vi "信号光谱11.vi"() -> ()   [LabVIEW 2018]
uses:
  <vilib>/Utility/NIReport.llb/Report Type.ctl
  <vilib>/Utility/file.llb/Write Delimited Spreadsheet (DBL).vi
  <vilib>/Instr/_visa.llb/VISA Configure Serial Port (Instr).vi
  <vilib>/addons/_office/excel.llb/Excel Get Data ([str]).vi
  <vilib>/Utility/NIReport.llb/NI_report.lvclass
  <vilib>/Analysis/NI_AALBase.lvlib
  <vilib>/ptbypt/NI_PtbyPt.lvlib
  <vilib>/Utility/NIReport.llb/NI_ReportGenerationCore.lvlib
  <vilib>/addons/_office/NI_ReportGenerationToolkit.lvlib
  <vilib>/Utility/NIReport.llb/Excel/NI_Excel.lvclass
panel:
  in  "Δy系数（0-1之间）":dbl=1.0 min=0.0 max=1.0
  in  "Δx系数（0-1之间）":dbl=1.0 min=0.0 max=1.0
  out "error out 2":errorcluster
  in  "y初次移动/um":dbl=2.0
  in  "y比例(步/um)":dbl=91.48
  in  "x比例(步/um)":dbl=91.48
  in  "x初次移动/um":dbl=2.0
  in  "运动加速度":i32=200
  in  "运动速度（步数/s）":i32=200
  out "y":i32
  out "x":i32
  out "DeviceKey Out":string
  out "Identification":string
  in  "画面长度（um）":dbl=41.52
  in  "截图等待时间（秒）":u32=10
  in  "y是否取反":bool
  in  "x是否取反":bool
  in  "是否移动光斑":bool
  out "波长范围":dbl[](array[numeric])
  out "Backlight":i32[][](graph)
  in  "?":enum32{"IHR 550", "CCD"}(tab)
  in  "Move To\nTarget Positions":bool
  out "Current UniqueID":string="Mono4"
  in  "Mono ID":string(combo)="Mono1"
  in  "Connect":bool
  out "Initialized JY":bool=TRUE
  in  "Force\nInitialization":bool
  in  "Target Grating":string(combo)="2"
  out "Current Description":string="1" caption="Description"
  out "Grating Index":i32=1
  out "Current Grating":dbl=1200.0
  out "Units":string="nm"
  out "Current WL":dbl=897.9988
  out "Exit Mirror\nPosition":i32(ring)=2 items=["EntranceMirror", "ExitMirror", "Front", "Side"]
  out "Entrance Mirror\nPosition":i32(ring)=2 items=["EntranceMirror", "ExitMirror", "Front", "Side"]
  out "Units 2":string="mm"
  out "Front Entrance":dbl
  in  "Target WL":dbl=2670.0
  in  "Exit Mirror":u16(ring)=3 caption="Target Position Exit Mirror" items=["Front"=2, "Side"=3]
  in  "Entrance Mirror":u16(ring)=2 caption="Target Position\nEntrance Mirror" items=["Front"=2, "Side"=3]
  in  "Target\nFront Entrance":dbl=1.0
  in  "Commande tab":T1(tab)
  in  "Area Number to Display":i32
  in  "Reformat":bool
  in  "GAIN":u16(ring)=2 caption="Device Name" items=["High Light", "Best Dynamic Range", "High Sensitivity"]
  in  "ADC":u16(ring) caption="Device Name" items=["20 kHz       ", " 1 MHz       ", " 1 MHz Ultra "]
  in  "Number of Areas :":u16=1 min=1 step=1
  in  "Integration time (ms) :":i16=30000
  out "Uniques ID":u16(ring) items=["CCD1", "CCD2"]
  in  "Device Name":u16(ring) items=["Synapse CCD (Lateral)", "Synapse_IGA (Axial)"]
  in  "Signal type :":enum16{"TTL Rising Edge", "TTL Falling Edge"}(ring)=enum."TTL Falling Edge"
  in  "Trigger Type :":u16(ring) items=["On Start"=1, "Per Acquisition"=2]
  in  "trigSigTypeString":string
  in  "trigEventString":string
  in  "Enable InputTriggers :":bool
  in  "Number of Cleans":i32=1
  in  "MultiAcqShutterMode":i32(ring)=3 items=["Open For All Spectra"=1, "Open for Each Spectrum"=3]
  in  "Accumulations:":u16=10 min=1 step=1
  in  "Multi Accumulation mode:":bool
  out "Y Pixels:":i32=256
  out "DataSize":i32=1024
  out "X Pixels:":i32=1024
  out "Firmware\nVersion":string="V1.20 CCD_4000"
  out "initialized ?":bool=TRUE
  in  "Continuous":bool
  in  "CCD Busy":bool
  out "indicator":string="Ready !"
  in  "initialize":bool
  in  "ShutterOpen":bool=TRUE caption="Shutter enable"
  in  "Acquire":bool
  in  "Temperature":bool
  in  "Setup":bool
  out "Acq Time(ms)":u32=3401
  in  "Save Backlight":bool
  in  "cut backlight":bool
  out "backlight":bool=TRUE
  in  "是否拟合":bool
  in  "是否保存":bool
  in  "停止程序":bool
  in  "上升下降沿/s":dbl format="%.2p"
  in  "延时/s":dbl format="%.2p"
  in  "占空比/%":dbl=3.0 format="%.2p"
  in  "高电平/V":dbl=4.0 format="%.2p"
  in  "频率/Hz":dbl=6000.0 format="%.3p"
  in  "低电平/V":dbl min=0.0 max=5.0 format="%.2p"
  out "configure error out":errorcluster
  in  "上升下降沿/s 2":dbl format="%.2p"
  in  "上升下降沿 2":i32(ring)=1 items=["上升沿", "下降沿"]
  in  "延时/s 2":dbl format="%.2p"
  in  "占空比/% 2":dbl=3.0 format="%.2p"
  in  "高电平/V 2":dbl=0.002 format="%.2p"
  in  "频率/Hz 2":dbl=6000.0 format="%.3p"
  in  "低电平/V 2":dbl min=0.0 max=5.0 format="%.2p"
  in  "输出信号波形 2":u16(ring) items=["Pulse"]
  in  "设置参数":bool
  out "output control error  4":errorcluster
  in  "低电平持续输出":bool
  in  "Enable":bool
  out "output control error  5":errorcluster
  out "output control error":errorcluster
  out "照明光error out":errorcluster
  in  "照明光VISA":refnum<visa-resource-name>="COM7"
  in  "baud rate":u32=9600 caption="baud rate (115200)" min=9600 max=115200
  in  "data bits (8)":u16=8 min=5 max=8 step=1
  in  "parity (0:none)":enum16{"None", "Odd", "Even", "Mark", "Space"}(ring)
  in  "stop bits (10: 1 bit)":u16(ring)=10 items=["1.0"=10, "1.5"=15, "2.0"=20]
  out "Δw2>C":bool=TRUE
  in  "C=w-w0":dbl=2.0 format="%#_13g"
  out "θi":dbl
  out "Δw1>C":bool=TRUE
  in  "角度倍乘系数":dbl=1.5
  in  "w0":dbl format="%#_13g"
  out "Spectrum":cluster{"Y":dbl[], "Y":dbl[]}[](graph)
  out "拟合参数":dbl[](array[numeric])
  out "xc":dbl
  out "w":dbl
  out "范围内？":bool[](array[boolean])
  in  "滤波阈值":dbl=3000.0 format="%#_13g"
  out "最终存储路径":path
  out "angle":dbl
  out "图片地址":string
  in  "开光时间/ms":u32=50
  out "正在测量":bool
  in  "终止测量":bool
  out "结果展示":dbl[][](array[numeric])=[[37.33100777239877, 2672.955043835526, 29.54153292599307, 222755.0, 50.0], [37.36593979472361, 2672.656498058864, 30.113284142729572, 222833.0, 50.0], [38.96986225690859, 2673.3337152325566, 33.38805102415213, 222910.0, 75.0], [37.39946104045098, 2676.4005085744548, 31.215565446104666, 222948.0, 47.0], [35.862209164247574, 2671.7826876859012, 30.355582265151796, 223028.0, 47.0]]
  in  "测量次数":i32=1
  in  "开始测量":bool
  in  "照明光":bool
  in  "Enable 2":bool
  out "Output 2":bool
  in  "上升下降沿":i32(ring)=1 items=["上升沿", "下降沿"]
  in  "channel输出口":i32(ring) items=["Channel 1", "Channel 2"]
  in  "输出信号波形":u16(ring) items=["Pulse"]
  out "output control error 2":errorcluster
  out "Output":bool
  in  "VISA 信号发生器":refnum<visa-resource-name>="USB0::0x1AB1::0x0641::DG4E192200870::INSTR"
  out "error out":errorcluster
  out "Gratings":dbl[](array[numeric])=[1200.0, 300.0]
  out "Data":i32[][](graph)
  out "trigAddress":i32
  out "Gain Number":i32[](array[numeric])=[10, 11, 12, 13, 8, 2]
  out "ADC Number":i32[](array[numeric])=[0, 1, 2, 3, 4]
  out "temp graph":dbl(graph)=-134.538067
  in  "Close":bool=TRUE
  out "JYCCDLib.IJYCCDReqd":refnum<k7>
  out "areas :":i32[][](array[numeric])=[[1], [1], [1], [1024], [256], [1], [256]]
  out "best fit":cluster{"Y":dbl[], "Y":dbl[]}[](graph)
  in  "拟合起点":i32=200
  in  "拟合终点":i32=850
  out "最终存储路径 2":path
  in  "Constante de condition\n(Voir l'aide contextuelle)":bool
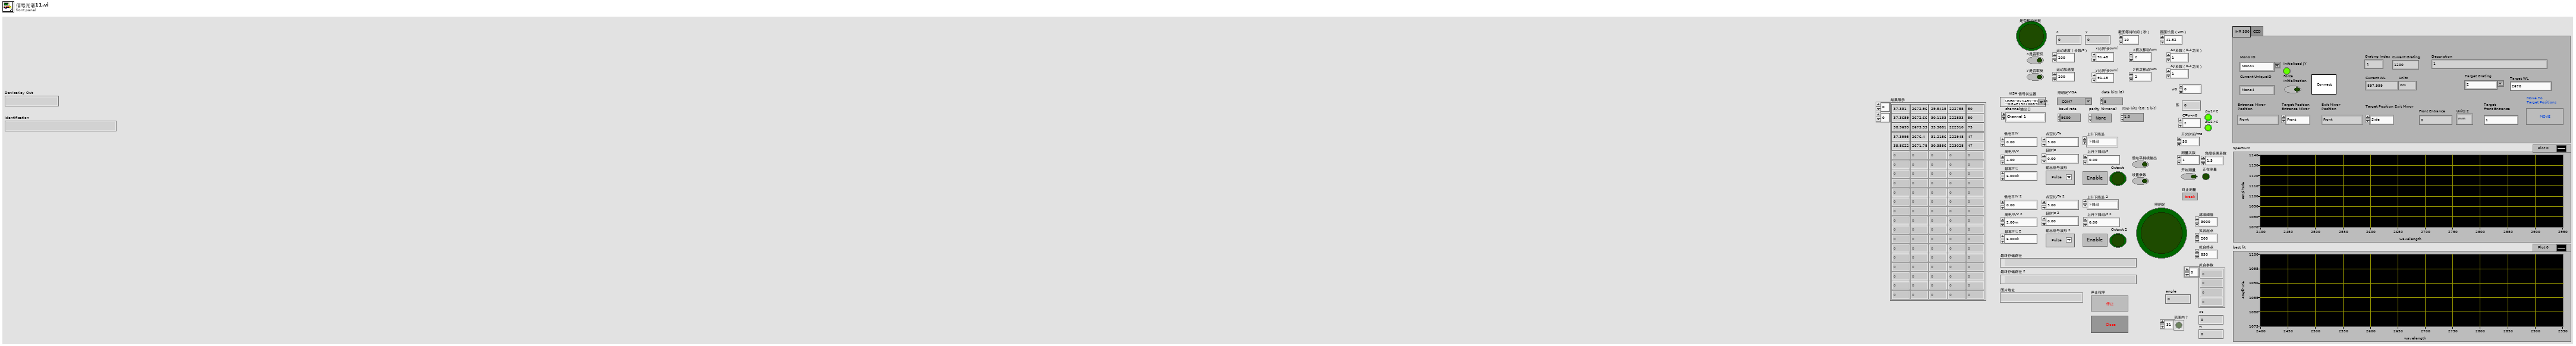
[diagram p1: front panel]
types:
  T1 = enum32{"Settings", "Trigger In", "Multi-Accu.", "Infos"}
  T2 = enum8{"Enabled", "Disabled", "Disabled and Grayed Out"}
  T3 = enum16{"maximized", "minimized", "normal", "no change"}
  T4 = typedef "NI_ReportGenerationCore.lvlib/Report Type.ctl" = enum16{"HTML", "Word", "Excel"}
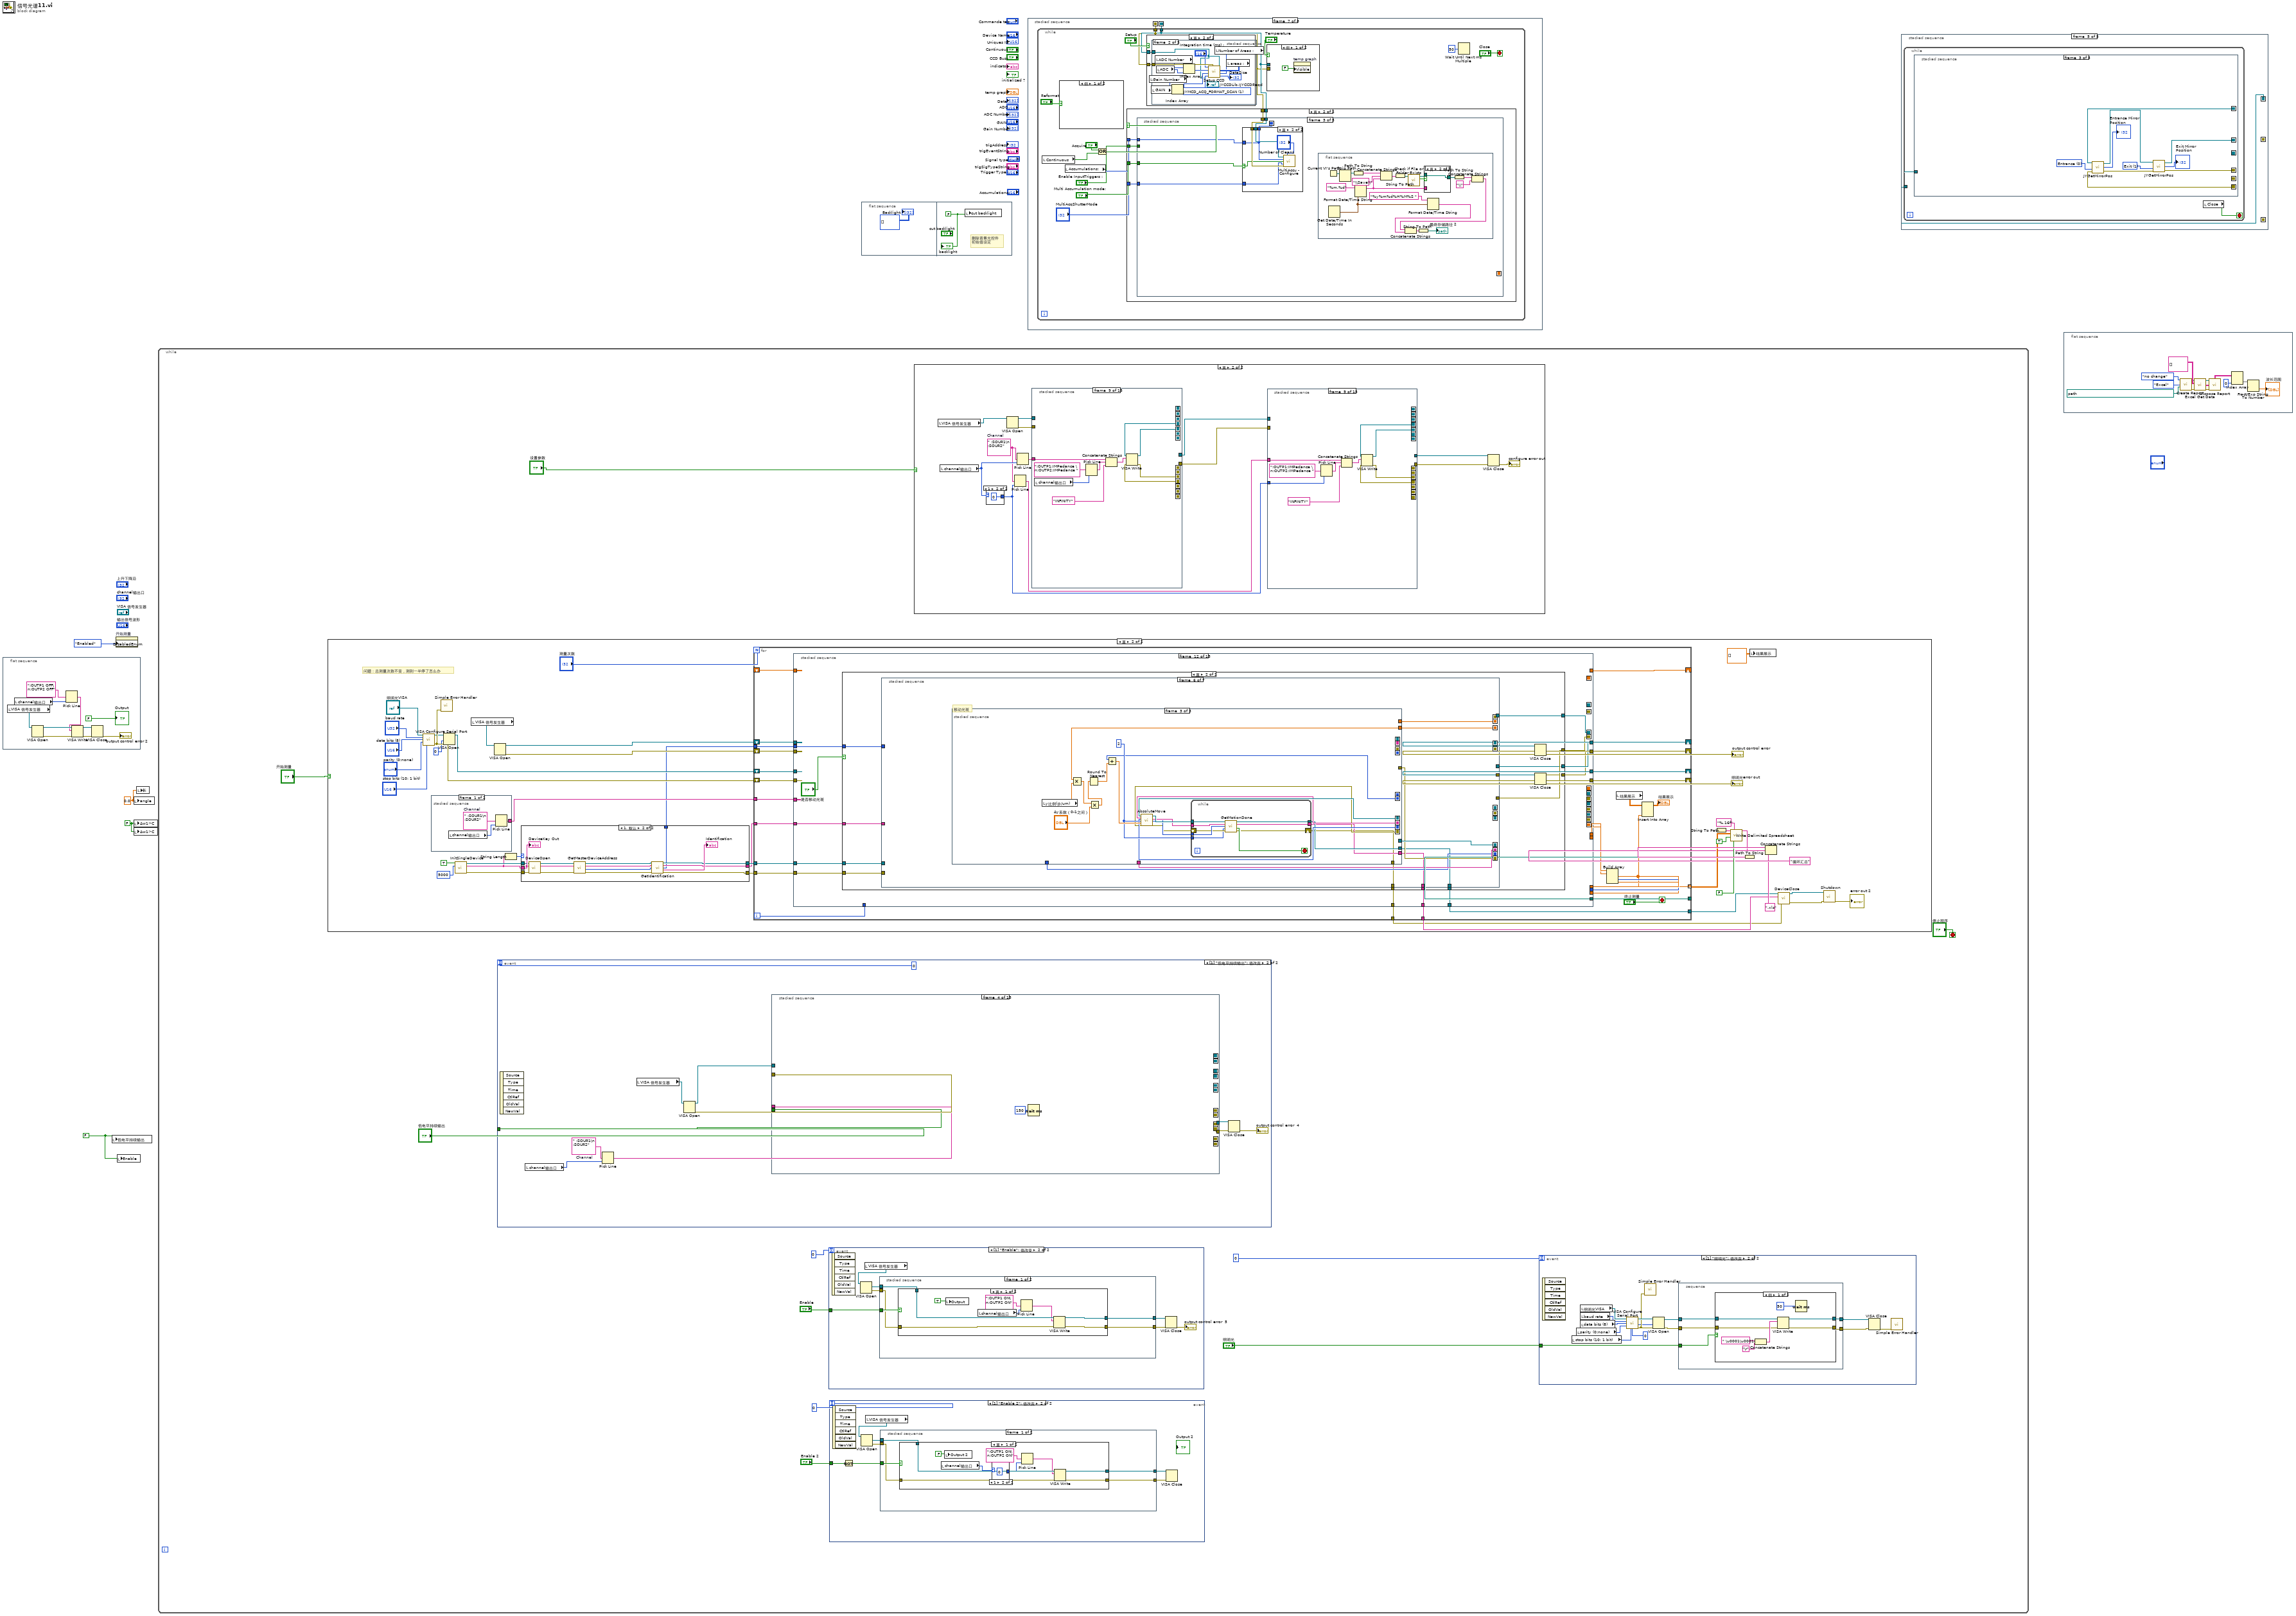
[diagram p0: block diagram]
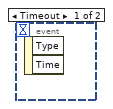
[diagram p2: hidden frame]
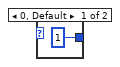
[diagram p3: hidden frame]
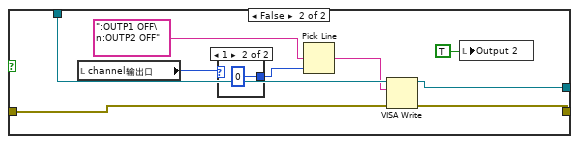
[diagram p4: hidden frame]
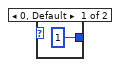
[diagram p5: hidden frame]
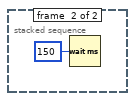
[diagram p6: hidden frame]
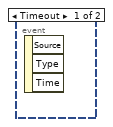
[diagram p7: hidden frame]
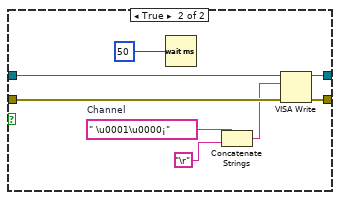
[diagram p8: hidden frame]
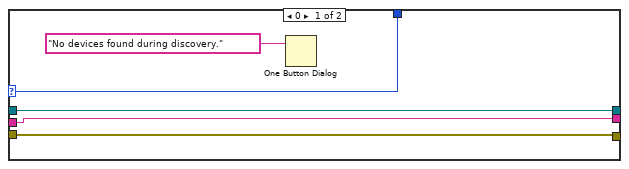
[diagram p10: hidden frame]
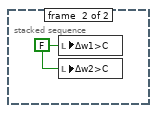
[diagram p11: hidden frame]
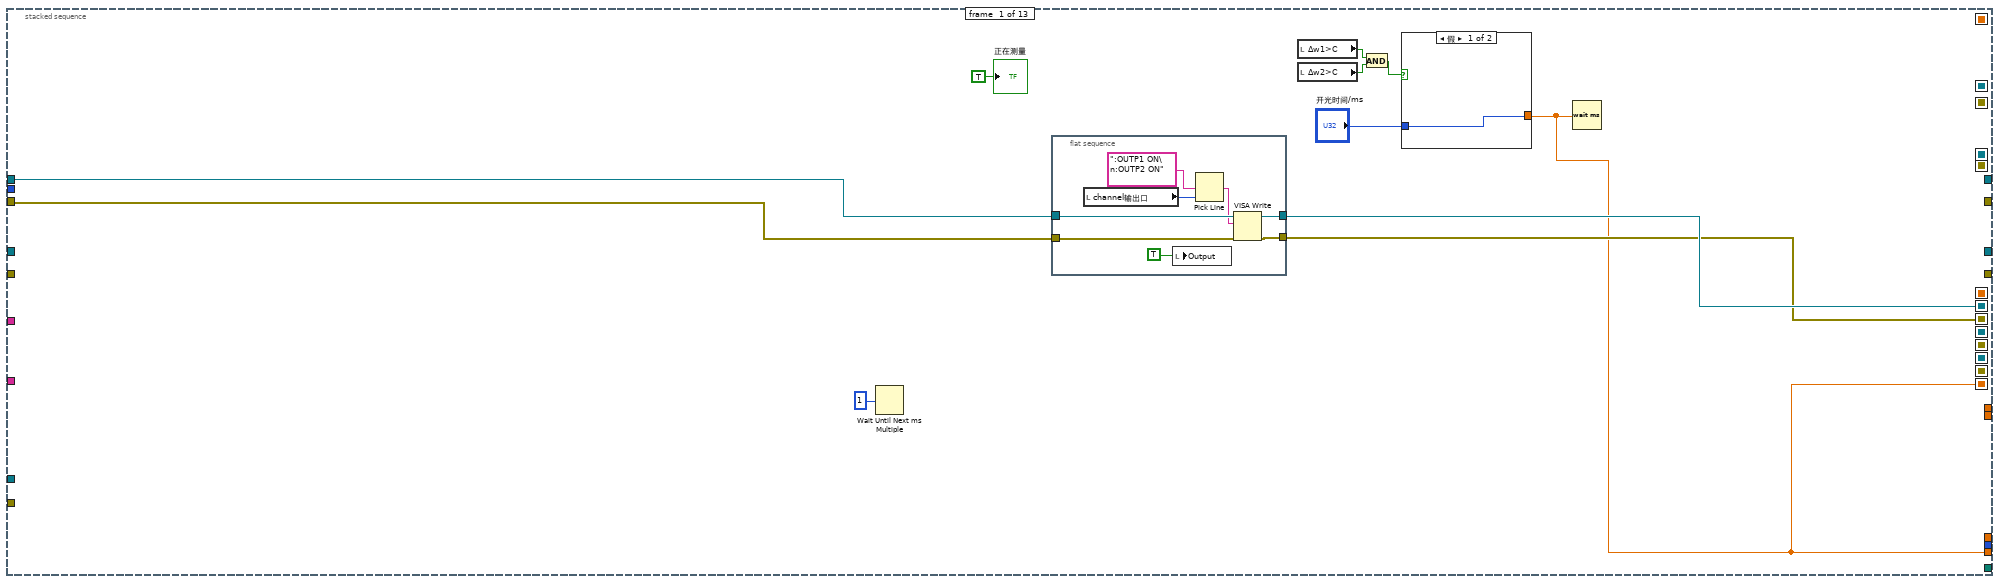
[diagram p12: hidden frame]
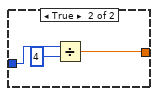
[diagram p13: hidden frame]
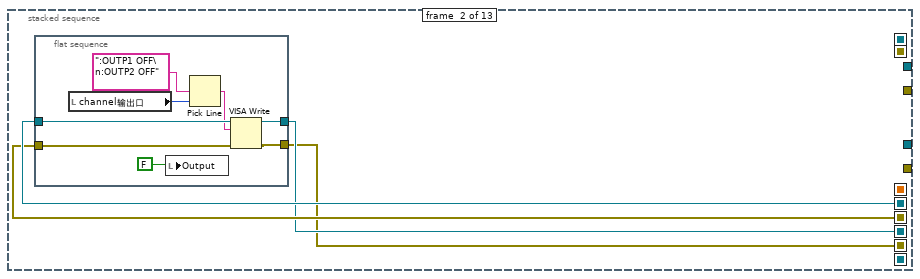
[diagram p14: hidden frame]
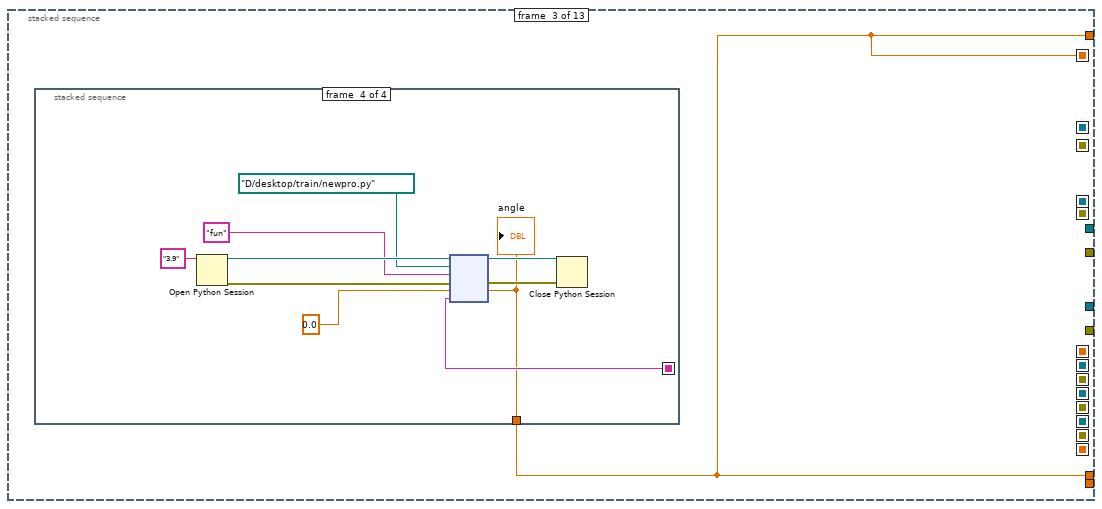
[diagram p15: hidden frame]
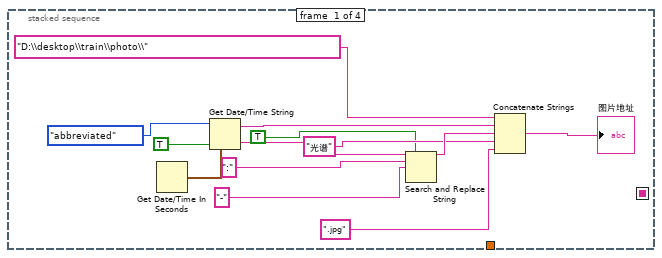
[diagram p16: hidden frame]
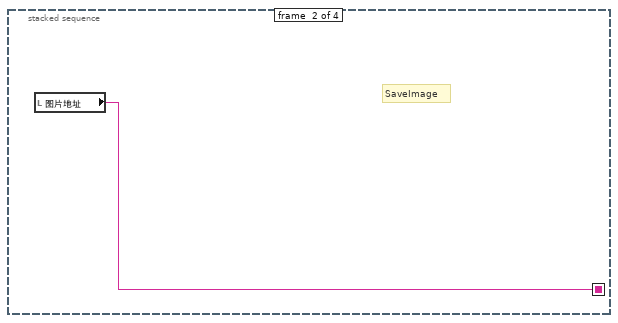
[diagram p17: hidden frame]
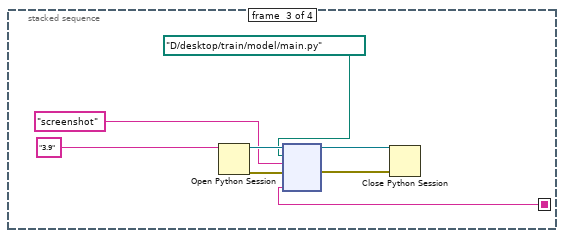
[diagram p18: hidden frame]
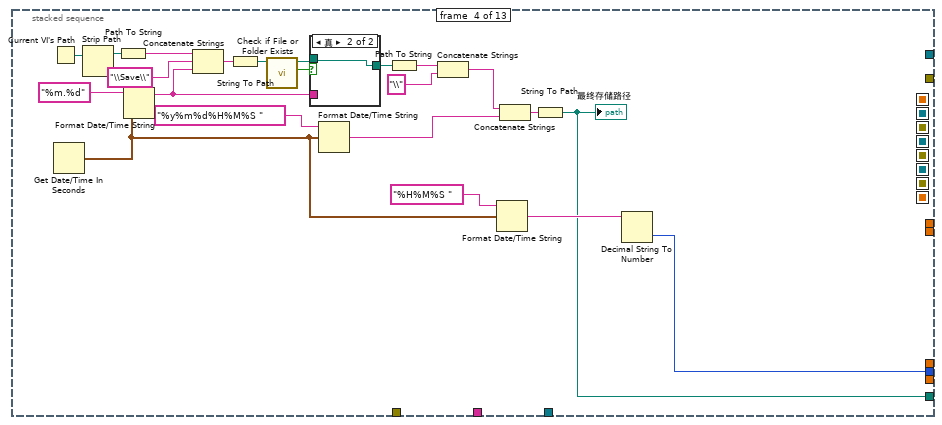
[diagram p19: hidden frame]
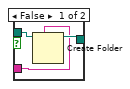
[diagram p20: hidden frame]
diagram:
  w2 = FALSE ("Δw1>C")
  w3 = 0.0 ("angle")
  w1 = FALSE
  n1 = flat-sequence {
    frame #0 {
      n2 = local read "VISA 信号发生器"() -> (w8:refnum<visa-resource-name>)
      n3 = local read "channel输出口"() -> (w6:i32)
      n4 = VISA Open(VISA resource name=w8) -> (VISA resource name=w14:refnum<visa-resource-name>, error out=w13:errorcluster)  [unwired: 4 in]
      n5 = Pick Line(multi-line string=":OUTP1 OFF\n:OUTP2 OFF" ("write buffer"), line index=w6) -> (output string=w5:string)  [unwired: 1 in]
      n6 = VISA Write(VISA resource name=w14, write buffer=w5, error in (no error)=w13) -> (VISA resource name out=w11:refnum<visa-resource-name>, error out=w10:errorcluster)  [unwired: 1 out]
      n7 = VISA Close(VISA resource name=w11, error in (no error)=w10) -> (error out=→"output control error 2":errorcluster)
      "Output" <- FALSE ("布尔")
    }
  }
  n8 = local write "低电平持续输出"(w1) -> ()
  n9 = property on="开始测量" class="Bool"("DisabledEnum"=T2."Enabled" ("禁用")) -> ()  [unwired: 2 in, 2 out]
  n10 = local write "Enable"(w1) -> ()
  n11 = local write "angle"(w3) -> ()
  n12 = local write "Δw1>C"(w2) -> ()
  n13 = local write "Δw1>C"(w2) -> ()
  n14 = local write "θi"(w3) -> ()
  n15 = while {
    stop <- "停止程序" stop-if-true
    n16 = case shown="真" "开始测量" {
      frame False {
      }
      frame True {
        # "问题：总测量次数不变，测到一半停了怎么办"
        n17 = call-poly "VISA Configure Serial Port"("VISA resource name"="照明光VISA", "baud rate (9600)"="baud rate", "data bits (8)"="data bits (8)", "parity (0:none)"="parity (0:none)", "stop bits (10: 1 bit)"="stop bits (10: 1 bit)") -> ("VISA resource name out"=w134:refnum<visa-resource-name>, "error out"=w135:errorcluster)  [unwired: 9 in]
        n18 = stacked-sequence {
          tunnel: [w164 _] -> w138
          frame #0 {
            w165 = " :SOUR1\n :SOUR2"  # Channel
            n19 = local read "channel输出口"() -> (w166:i32)
            n20 = Pick Line(multi-line string=w165, line index=w166) -> (output string=w164:string)  [unwired: 1 in]
          }
          frame #1 {
            w167 = FALSE ("Δw1>C")
            n21 = local write "Δw1>C"(w167) -> ()
            n22 = local write "Δw2>C"(w167) -> ()
          }
        }
        n23 = call <vilib>:"Simple Error Handler.vi"("error in (no error)"=w135) -> ()  [unwired: 4 in, 5 out]
        n24 = VISA Open(access mode=0, error in (no error)=w135, VISA resource name=w134) -> (VISA resource name=w127:refnum<visa-resource-name>, error out=w126:errorcluster)  [unwired: 2 in]
        n25 = call "InitSingleDevice.vi"("msecDelayForDiscovery"=5000, "logging"=TRUE) -> ("error out"=w107:errorcluster, "DeviceKey Out"=w106:string, "CmdLib Out"=w108:refnum<k24>)  [unwired: 3 in]
        n26 = local read "VISA 信号发生器"() -> (w143:refnum<visa-resource-name>)
        n27 = VISA Open(VISA resource name=w143) -> (VISA resource name=w142:refnum<visa-resource-name>, error out=w141:errorcluster)  [unwired: 4 in]
        n28 = String Length(string=w106) -> (length=w109:i32)
        n29 = case shown="1, 默认" w109 {
          selector: w109 -> [w144 _]
          tunnel: w108 -> [w147 w154]
          tunnel: w107 -> [w146 w158]
          tunnel: w106 -> [w145 w156]
          tunnel: [w147 w152] -> w105
          tunnel: [w146 w151] -> w103
          tunnel: [w145 w150] -> w104
          tunnel: [w144 w149] -> w102
          frame 0 {
            n30 = One Button Dialog(message="No devices found during discovery.") -> ()  [unwired: 1 in, 1 out]
          }
          frame 1, Default {
            n31 = call "DeviceOpen.vi"("error in (no error)"=w158, "DeviceKey In"=w156, "CmdLib In"=w154) -> ("error out"=w157:errorcluster, "DeviceKey Out"=w155:string, "CmdLib Out"=w153:refnum<k24>)  [unwired: 2 in]
            n32 = call "GetMasterDeviceAddress.vi"("error in (no error)"=w157, "DeviceKey In"=w155, "CmdLib In"=w153) -> ("error out"=w161:errorcluster, "Device Address"=w162:i32, "DeviceKey Out"=w159:string, "CmdLib Out"=w160:refnum<k24>)  [unwired: 1 in]
            n33 = call "GetIdentification.vi"("CmdLib In"=w160, "DeviceKey In"=w159, "Device Address In"=w162, "error in (no error)"=w161) -> ("CmdLib Out"=w152:refnum<k24>, "DeviceKey Out"=w150:string, "Device Address Out"=w149:i32, "Identification"=→"Identification":string, "error out"=w151:errorcluster)  [unwired: 7 in]
            "DeviceKey Out" <- w156
          }
        }
        n34 = for {
          N: "测量次数" -> [_]
          tunnel: w138 -> [w194]
          shift-right: [w190] -> w137
          shift-left: w142 -> [w196]
          shift-right: [w189] -> w136
          shift-left: w141 -> [w195]
          shift-right: [w188] -> w140
          shift-left: w127 -> [w193]
          shift-right: [w187] -> w139
          shift-left: w126 -> [w192]
          tunnel: [w177] -> w116 mode=indexing
          shift-right: [w182] -> _
          shift-left: _ -> [w181]
          tunnel: [w178] -> w113
          tunnel: w105 -> [w174]
          tunnel: w104 -> [w173]
          tunnel: w103 -> [w172]
          tunnel: w102 -> [w171]
          tunnel: [w170] -> w101
          tunnel: [w169] -> w100
          tunnel: [w168] -> w99
          i -> [w180]
          stop <- "终止测量" stop-if-true
          n35 = stacked-sequence {
            seq-local: [w203 _ _ _ _ _ _ _ _ _ _ _ _] -> [_ w223 _ _ _ _ _ _ _ _ _ _ _]
            seq-local: [w202 _ _ _ _ _ _ _ _ _ _ _ _] -> [_ w222 _ _ _ _ _ _ _ _ _ _ _]
            seq-local: [_ _ _ _ _ w308 _ _ _ _ _ _ _] -> [_ _ _ _ _ _ _ _ w426 _ _ _ _]
            seq-local: [_ _ _ _ _ w307 _ _ _ _ _ _ _] -> [_ _ _ _ _ _ _ _ w427 _ _ _ _]
            seq-local: [_ w221 _ _ _ _ _ _ _ _ _ _ _] -> [_ _ _ _ w294 _ _ _ _ _ _ _ _]
            seq-local: [_ w220 _ _ _ _ _ _ _ _ _ _ _] -> [_ _ _ _ w293 _ _ _ _ _ _ _ _]
            seq-local: [_ _ _ _ w292 _ _ _ _ _ _ _ _] -> [_ _ _ _ _ _ _ w410 _ _ _ _ _]
            seq-local: [_ _ _ _ w291 _ _ _ _ _ _ _ _] -> [_ _ _ _ _ _ _ w409 _ _ _ _ _]
            seq-local: [_ _ w232 _ _ _ _ _ _ _ _ _ _] -> [_ _ _ _ _ _ _ _ _ _ w436 _ _]
            seq-local: [_ _ _ _ _ _ w317 _ _ _ _ _ _] -> [_ _ _ _ _ _ _ _ _ _ w431 _ _]
            seq-local: [w197 _ _ _ _ _ _ _ _ _ _ _ _] -> [_ _ _ _ _ _ w315 _ _ _ _ _ _]
            seq-local: [_ _ _ _ _ _ _ w407 _ _ _ _ _] -> [_ _ _ _ _ _ _ _ _ _ _ w505 _]
            seq-local: [_ _ _ _ _ _ _ w408 _ _ _ _ _] -> [_ _ _ _ _ _ _ _ _ _ _ w504 _]
            tunnel: w196 -> [w205 _ _ _ _ _ _ _ _ _ _ _ _]
            tunnel: w195 -> [w204 _ _ _ _ _ _ _ _ _ _ _ _]
            tunnel: [_ _ _ _ _ _ _ _ _ _ _ w503 _] -> w190
            tunnel: [_ _ _ _ _ _ _ _ _ _ _ w502 _] -> w189
            tunnel: w194 -> [_ _ _ _ _ _ _ _ _ _ _ _ _]
            tunnel: w193 -> [_ _ _ _ _ w311 _ _ _ _ _ _ _]
            tunnel: w192 -> [_ _ _ _ _ w310 _ _ _ _ _ _ _]
            tunnel: [_ _ _ _ _ _ _ _ w423 _ _ _ _] -> w188
            tunnel: [_ _ _ _ _ _ _ _ w422 _ _ _ _] -> w187
            tunnel: [_ _ w232 _ _ _ _ _ _ _ _ _ _] -> w186
            tunnel: [_ _ _ _ _ _ w318 _ _ _ _ _ _] -> w185
            tunnel: [_ _ _ _ _ _ w317 _ _ _ _ _ _] -> w184
            tunnel: [_ _ _ w266 _ _ _ _ _ _ _ _ _] -> w183
            tunnel: [w197 _ _ _ _ _ _ _ _ _ _ _ _] -> w179
            tunnel: [_ _ w232 _ _ _ _ _ _ _ _ _ _] -> w182
            tunnel: w181 -> [_ _ _ _ _ _ _ _ _ _ w435 _ _]
            tunnel: w180 -> [_ _ _ _ _ _ _ _ _ _ w433 _ _]
            tunnel: [_ _ _ w265 _ _ _ _ _ _ _ _ _] -> w178
            tunnel: w174 -> [_ _ _ _ _ _ _ _ _ _ _ w501 _]
            tunnel: w173 -> [_ _ _ _ _ _ _ _ _ _ _ w500 _]
            tunnel: w172 -> [_ _ _ _ _ _ _ _ _ _ _ w499 _]
            tunnel: w171 -> [_ _ _ _ _ _ _ _ _ _ _ w498 _]
            tunnel: [_ _ _ _ _ _ _ _ _ _ _ w497 _] -> w170
            tunnel: [_ _ _ _ _ _ _ _ _ _ _ w496 _] -> w169
            tunnel: [_ _ _ _ _ _ _ _ _ _ _ w495 _] -> w168
            frame #0 {
              n36 = Wait Until Next ms Multiple(millisecond multiple=u32 1 ("毫秒倍数")) -> ()  [unwired: 1 out]
              n37 = flat-sequence {
                tunnel: w205 -> [w219]
                tunnel: w204 -> [w218]
                tunnel: [w213] -> w203
                tunnel: [w212] -> w202
                frame #0 {
                  n38 = local read "channel输出口"() -> (w215:i32)
                  n39 = local write "Output"(TRUE ("布尔")) -> ()
                  n40 = Pick Line(multi-line string=":OUTP1 ON\n:OUTP2 ON" ("write buffer"), line index=w215) -> (output string=w214:string)  [unwired: 1 in]
                  n41 = VISA Write(VISA resource name=w219, write buffer=w214, error in (no error)=w218) -> (VISA resource name out=w213:refnum<visa-resource-name>, error out=w212:errorcluster)  [unwired: 1 out]
                }
              }
              n42 = local read "Δw1>C"() -> (w199:bool)
              n43 = local read "Δw2>C"() -> (w200:bool)
              n44 = And(x=w199, y=w200) -> (x .and. y?=w198:bool)
              n45 = case shown="假" w198 {
                tunnel: [w208 w209] -> w197
                tunnel: "开光时间/ms" -> [w208 w211]
                frame False {
                }
                frame True {
                  n46 = Divide(x=w211, y=u32 4) -> (x/y=w209:dbl)
                }
              }
              n47 = Wait (ms)(milliseconds to wait=w197) -> ()  [unwired: 1 out]
              "正在测量" <- TRUE
            }
            frame #1 {
              n48 = flat-sequence {
                tunnel: w223 -> [w231]
                tunnel: w222 -> [w230]
                tunnel: [w225] -> w221
                tunnel: [w224] -> w220
                frame #0 {
                  n49 = local read "channel输出口"() -> (w227:i32)
                  n50 = local write "Output"(FALSE ("布尔")) -> ()
                  n51 = Pick Line(multi-line string=":OUTP1 OFF\n:OUTP2 OFF" ("write buffer"), line index=w227) -> (output string=w226:string)  [unwired: 1 in]
                  n52 = VISA Write(VISA resource name=w231, write buffer=w226, error in (no error)=w230) -> (VISA resource name out=w225:refnum<visa-resource-name>, error out=w224:errorcluster)  [unwired: 1 out]
                }
              }
            }
            frame #2 {
              n53 = stacked-sequence {
                seq-local: [_ w246 _ _] -> [_ _ w247 w256]
                tunnel: [_ _ _ w255] -> w232
                frame #0 {
                  n54 = Get Date/Time In Seconds() -> (seconds since 1Jan1904=w242:timestamp)
                  n55 = Get Date/Time String(date format (0)=enum16{"short", "long", "abbreviated"}."abbreviated" ("日期格式(0)"), seconds (now)=w242, want seconds? (F)=TRUE ("需要秒？(F)")) -> (date string=w245:string, time string=w243:string)
                  n56 = Search and Replace String(replace all?=TRUE ("替换全部？(F)"), input string=w243, search string=":" ("搜索字符串"), replace string="-" ("替换字符串(\"\")")) -> (result string=w244:string)  [unwired: 4 in, 3 out]
                  n57 = Concatenate Strings("D:\\desktop\\train\\photo\\", w245, w244, "光谱" ("字符串"), ".jpg" ("字符串")) -> (→"图片地址":string)
                }
                frame #1 {
                  # "SaveImage"
                  n58 = local read "图片地址"() -> (w246:string)
                }
                frame #2 {
                  n59 = Open Python Session(python version="3.9" ("Python version")) -> (session out=w254:refnum<k35>, error out=w252:errorcluster)  [unwired: 2 in]
                  n60 = node(w254, path "D:/desktop/train/model/main.py" ("module path"), "screenshot" ("function name"), w252, w247) -> (w253:refnum<k35>, w251:errorcluster)  [unwired: 3 in, 2 out]
                  n61 = Close Python Session(session in=w253, error in=w251) -> ()  [unwired: 1 out]
                }
                frame #3 {
                  n62 = Open Python Session(python version="3.9" ("Python version")) -> (session out=w263:refnum<k35>, error out=w261:errorcluster)  [unwired: 2 in]
                  n63 = node(w263, path "D:/desktop/train/newpro.py" ("module path"), "fun" ("function name"), w261, 0.0, w256) -> (w262:refnum<k35>, w260:errorcluster, w255:dbl)  [unwired: 1 in, 2 out]
                  "angle" <- w255
                  n64 = Close Python Session(session in=w262, error in=w260) -> ()  [unwired: 1 out]
                }
              }
            }
            frame #3 {
              n65 = Current VI's Path() -> (path=w275:path)
              n66 = Get Date/Time In Seconds() -> (seconds since 1Jan1904=w268:timestamp)
              n67 = Strip Path(path=w275) -> (stripped path=w276:path)  [unwired: 1 out]
              n68 = Path To String(path=w276) -> (string=w277:string)
              n69 = Format Date/Time String(time format string (%c)="%m.%d" ("时间格式字符串(%c)"), seconds (now)=w268) -> (date/time string=w283:string)  [unwired: 1 in]
              n70 = Concatenate Strings(w277, "\\Save\\" ("字符串"), w283) -> (w278:string)
              n71 = String To Path(string=w278) -> (path=w279:path)
              n72 = call <vilib>:"Check if File or Folder Exists.vi"("path"=w279) -> ("file or folder exists?"=w280:bool, "dup path"=w282:path)  [unwired: 8 in, 1 out]
              n73 = case shown="真" w280 {
                tunnel: [w289 w290] -> w281
                tunnel: w282 -> [w288 w290]
                tunnel: w283 -> [w287 _]
                frame False {
                  n74 = Create Folder(prompt (Create Folder)=w287, path (use dialog)=w288) -> (created path=w289:path)  [unwired: 1 in, 2 out]
                }
                frame True {
                }
              }
              n75 = Format Date/Time String(time format string (%c)="%y%m%d%H%M%S " ("时间格式字符串(%c)"), seconds (now)=w268) -> (date/time string=w286:string)  [unwired: 1 in]
              n76 = Path To String(path=w281) -> (string=w284:string)
              n77 = Concatenate Strings(w284, "\\" ("字符串")) -> (w285:string)
              n78 = Format Date/Time String(time format string (%c)="%H%M%S " ("时间格式字符串(%c)"), seconds (now)=w268) -> (date/time string=w267:string)  [unwired: 1 in]
              n79 = Concatenate Strings(w285, w286) -> (w274:string)
              n80 = String To Path(string=w274) -> (path=w265:path)
              "最终存储路径" <- w265
              n81 = Decimal String To Number(string=w267) -> (number=w266:i32)  [unwired: 2 in, 1 out]
            }
            frame #4 {
              n82 = flat-sequence {
                tunnel: w294 -> [w303]
                tunnel: w293 -> [w302]
                tunnel: [w298] -> w292
                tunnel: [w297] -> w291
                frame #0 {
                  n83 = local read "channel输出口"() -> (w296:i32)
                  n84 = case shown="1" w296 {
                    tunnel: [1 0] -> w295
                    frame 0, Default {
                    }
                    frame 1 {
                    }
                  }
                  n85 = local write "Output 2"(FALSE ("布尔")) -> ()
                  n86 = Pick Line(multi-line string=":OUTP1 OFF\n:OUTP2 OFF" ("write buffer"), line index=w295) -> (output string=w299:string)  [unwired: 1 in]
                  n87 = VISA Write(VISA resource name=w303, write buffer=w299, error in (no error)=w302) -> (VISA resource name out=w298:refnum<visa-resource-name>, error out=w297:errorcluster)  [unwired: 1 out]
                }
              }
            }
            frame #5 {
              w306 = " \u0001\u0001¢"  # Channel
              n88 = Wait (ms)(milliseconds to wait=500) -> ()  [unwired: 1 out]
              n89 = Concatenate Strings(w306, "\r") -> (w312:string)
              n90 = local write "照明光"(FALSE ("照明光")) -> ()
              n91 = VISA Write(VISA resource name=w311, write buffer=w312, error in (no error)=w310) -> (VISA resource name out=w308:refnum<visa-resource-name>, error out=w307:errorcluster)  [unwired: 1 out]
            }
            frame #6 {
              n92 = local read "Area Number to Display"() -> (w360:i32)
              n93 = local read "JYCCDLib.IJYCCDReqd"() -> (w356:refnum<k7>)
              n94 = Get Date/Time In Seconds() -> (seconds since 1Jan1904=w369:timestamp)
              n95 = local read "最终存储路径"() -> (w383:path)
              n96 = Get Date/Time String(date format (0)=enum16{"short", "long", "abbreviated"}."abbreviated" ("日期格式(0)"), seconds (now)=w369, want seconds? (F)=TRUE ("需要秒？(F)")) -> (date string=w377:string, time string=w372:string)
              n97 = call "MultiAccu - Acquire spectral.vi"("error in"=errorcluster {"status"=FALSE, "code"=0, "source"=""}, "Accumulations:"=u16 1, "ShutterOpen"=TRUE, "JYCCDLib.IJYCCDReqd"=w356) -> ("Acq Time(ms)"=w362:u32, "Array Out"=w361:i32[][][])  [unwired: 1 out]
              n98 = local write "Acq Time(ms)"(w362) -> ()
              n99 = local read "cut backlight"() -> (w344:bool)
              n100 = local read "backlight"() -> (w342:bool)
              n101 = Search and Replace String(replace all?=TRUE ("替换全部？(F)"), input string=w372, search string=":" ("搜索字符串"), replace string="-" ("替换字符串(\"\")")) -> (result string=w376:string)  [unwired: 4 in, 3 out]
              n102 = Path To String(path=w383) -> (string=w366:string)
              n103 = And(x=w344, y=w342) -> (x .and. y?=w343:bool)
              n104 = call "Array reset dimension.vi"("Area Number"=w360, "Array In"=w361) -> ("Array Out"=w346:i32[][])
              n105 = Concatenate Strings(w366, w377, w376, "光谱" ("字符串"), ".xls" ("字符串")) -> (w381:string)
              n106 = case shown="真" w343 {
                tunnel: [w403 w405] -> w345
                tunnel: w346 -> [w403 w404]
                frame False {
                }
                frame True {
                  n107 = local read "Backlight"() -> (w406:i32[][])
                  n108 = Subtract(x=w404, y=w406) -> (x-y=w405:i32[][])
                }
              }
              n109 = String To Path(string=w381) -> (path=w382:path)
              n110 = local write "Data"(w346) -> ()
              n111 = local read "波长范围"() -> (w323:dbl[])
              n112 = Index Array(array=w345, index (row)=0 ("索引 (行)")) -> (element=w384:i32[])  [unwired: 1 in]
              n113 = Reverse 1D Array(array=w384) -> (reversed array=w320:i32[])
              n114 = local read "angle"() -> (w322:dbl)
              n115 = local read "拟合起点"() -> (w332:i32)
              n116 = local read "拟合终点"() -> (w334:i32)
              n117 = call <vilib>:"Median Filter.vi"("left rank"=6, "X"=w320) -> ("Filtered X"=w319:dbl[])  [unwired: 8 in, 1 out]
              n118 = Build Array(w322, w315, 0.0 ("元素")) -> (w321:dbl[])
              n119 = Subtract(x=w334, y=w332) -> (x-y=w331:i32)
              n120 = call "Convert to Dynamic Data"("Array"=w323) -> ("Dynamic Data Type"=w353:dynamicdata)  [unwired: 3 in]
              n121 = call "Convert to Dynamic Data2"("Array"=w320) -> ("Dynamic Data Type"=w352:dynamicdata)  [unwired: 3 in]
              n122 = Array Subset(array=w323, index=w332, length=w331) -> (w329:dbl[])
              n123 = call "Build XY Graph2"("Y Input"=w352, "X Input"=w353) -> ("XY Graph"=→"Spectrum":cluster{"Y":dbl[], "Y":dbl[]}[])  [unwired: 8 in, 1 out]
              n124 = call "转换至动态数据6"("Array"=w329) -> ("Dynamic Data Type"=w350:dynamicdata)  [unwired: 3 in]
              n125 = In Range and Coerce(upper limit="滤波阈值", x=w319, lower limit=-100.0) -> (In Range?=w337:bool[])  [unwired: 1 out]
              "范围内？" <- w337
              n126 = Not(x=w337) -> (.not. x?=w336:bool[])
              n127 = Or Array Elements(Boolean array=w336) -> (logical OR=w339:bool)
              n128 = local read "X Pixels:"() -> (w338:i32)
              n129 = local read "波长范围"() -> (w324:dbl[])
              n130 = local read "滤波阈值"() -> (w335:dbl)
              n131 = case shown="真" w339 {
                tunnel: w338 -> [_ w390]
                tunnel: w319 -> [w386 w389]
                tunnel: [w386 w388] -> w330
                tunnel: w335 -> [_ w387]
                frame False {
                }
                frame True {
                  n132 = for {
                    N: w390 -> [_]
                    tunnel: w389 -> [w394] mode=indexing
                    tunnel: [w393] -> w388 mode=indexing
                    shift-right: [w393] -> _
                    shift-left: _ -> [w392]
                    tunnel: w387 -> [w391]
                    n133 = Greater?(x=w394, y=w391) -> (0:w396:bool)
                    n134 = Less?(x=w394, y=-100.0) -> (x < y?=w397:bool)
                    n135 = Or(x=w396, y=w397) -> (x .or. y?=w395:bool)
                    n136 = case shown="真" w395 {
                      tunnel: w394 -> [w399 _]
                      tunnel: [w399 w401] -> w393
                      tunnel: w392 -> [_ w402]
                      frame False {
                      }
                      frame True {
                        n137 = call <vilib>:"Median Filter PtByPt.vi"("rank"=5, "x"=w402) -> ("Filtered x"=w401:dbl)  [unwired: 2 in, 1 out]
                      }
                    }
                  }
                }
              }
              n138 = Array Subset(array=w330, index=w332, length=w331) -> (w333:dbl[])
              n139 = call "转换至动态数据5"("Array"=w333) -> ("Dynamic Data Type"=w351:dynamicdata)  [unwired: 3 in]
              n140 = call "曲线拟合2"("Locations"=w350, "Signals"=w351) -> ("best fit"=w355:dynamicdata, "non-linear coefficients"=w354:dynamicdata)  [unwired: 5 in, 3 out]
              n141 = call "从动态数据转换3"("Dynamic Data Type"=w354) -> ("Array"=w347:dbl[])  [unwired: 3 in]
              "拟合参数" <- w347
              n142 = call "从动态数据转换4"("Dynamic Data Type"=w355) -> ("Array"=w328:dbl[])  [unwired: 3 in]
              n143 = Build Array(w323, w319, w328, w347, w321) -> (w385:dbl[][])
              n144 = call-poly <vilib>:"Write Delimited Spreadsheet.vi"("file path (dialog if empty)"=w382, "format (%.3f)"="%.16f", "2D data"=w385, "append to file? (new file:F)"=TRUE ("append to file? (F)"), "transpose? (no:F)"=TRUE ("transpose? (F)")) -> ()  [unwired: 9 in, 2 out]
              n145 = Index Array(array=w347, index #1=0 ("索引"), index #2=1 ("索引")) -> (element #1=w318:dbl, element #2=w317:dbl)
              "xc" <- w318
              "w" <- w317
              n146 = Bundle("波长范围"=w324, "Filtered X"=w330) -> (w327:cluster{"波长范围 ":dbl[], "Filtered X":dbl[]})  [unwired: 1 in]
              n147 = Bundle(w329, "Array"=w328) -> (w326:cluster{dbl[], "Array":dbl[]})  [unwired: 1 in]
              n148 = Build Array(w327, w326) -> (w325:cluster{"波长范围 ":dbl[], "Array":dbl[]}[])
              n149 = local write "best fit"(w325) -> ()
            }
            frame #7 {
              n150 = flat-sequence {
                tunnel: w410 -> [w419]
                tunnel: w409 -> [w418]
                tunnel: [w414] -> w407
                tunnel: [w413] -> w408
                frame #0 {
                  n151 = local read "channel输出口"() -> (w412:i32)
                  n152 = case shown="0, 默认" w412 {
                    tunnel: [1 0] -> w411
                    frame 0, Default {
                    }
                    frame 1 {
                    }
                  }
                  n153 = local write "Output 2"(TRUE ("布尔")) -> ()
                  n154 = Pick Line(multi-line string=":OUTP1 ON\n:OUTP2 ON" ("write buffer"), line index=w411) -> (output string=w415:string)  [unwired: 1 in]
                  n155 = VISA Write(VISA resource name=w419, write buffer=w415, error in (no error)=w418) -> (VISA resource name out=w414:refnum<visa-resource-name>, error out=w413:errorcluster)  [unwired: 1 out]
                }
              }
            }
            frame #8 {
              w424 = " \u0001\u0000¡"  # Channel
              n156 = Concatenate Strings(w424, "\r") -> (w428:string)
              n157 = VISA Write(VISA resource name=w426, write buffer=w428, error in (no error)=w427) -> (VISA resource name out=w423:refnum<visa-resource-name>, error out=w422:errorcluster)  [unwired: 1 out]
              n158 = local write "照明光"(TRUE ("照明光")) -> ()
            }
            frame #9 {
              n159 = Wait (ms)(milliseconds to wait=1200) -> ()  [unwired: 1 out]
            }
            frame #10 {
              n160 = Greater Or Equal?(x=w433, y=1) -> (x >= y?=w434:bool)
              n161 = case shown="假" w434 {
                tunnel: w436 -> [_ w442]
                tunnel: w435 -> [_ w443]
                tunnel: w431 -> [w437 w444]
                frame False {
                  n162 = local write "w0"(w437) -> ()
                }
                frame True {
                  n163 = local read "Δw1>C"() -> (w441:bool)
                  n164 = case shown="真" w441 {
                    tunnel: w444 -> [w463 w483]
                    tunnel: w443 -> [w453 _]
                    tunnel: w442 -> [w454 _]
                    frame False {
                      # "判断Δw突变位置并记录当前θ值"
                      # "根据θ变化速度改变开光时间"
                      n165 = local read "w0"() -> (w461:dbl)
                      n166 = Subtract(x=w454, y=w453) -> (x-y=w456:dbl)
                      n167 = local read "开光时间/ms"() -> (w459:u32)
                      n168 = Subtract(x=w461, y=w463) -> (x-y=w466:dbl)
                      n169 = Absolute Value(x=w456) -> (abs(x)=w458:dbl)
                      n170 = Absolute Value(x=w466) -> (abs(x)=w464:dbl)
                      n171 = Greater Or Equal?(x=w458, y=0.3) -> (x >= y?=w457:bool)
                      n172 = Greater Or Equal?(x=w464, y="C=w-w0") -> (x >= y?=w462:bool)
                      n173 = case shown="真" w462 {
                        tunnel: w453 -> [_ w481]
                        frame False {
                          w479 = FALSE ("Δw1>C")
                          n174 = local write "Δw1>C"(w479) -> ()
                          n175 = local write "Δw2>C"(w479) -> ()
                        }
                        frame True {
                          "θi" <- w481
                          "Δw1>C" <- TRUE ("布尔")
                        }
                      }
                      n176 = case shown="假" w457 {
                        tunnel: w458 -> [w471 _]
                        tunnel: w459 -> [w468 w478]
                        tunnel: [w467 w476] -> w460
                        frame False {
                          n177 = Less Or Equal?(x=w471, y=0.15) -> (x <= y?=w469:bool)
                          n178 = case shown="真" w469 {
                            tunnel: w468 -> [w472 w475]
                            tunnel: [w472 w474] -> w467
                            frame False {
                            }
                            frame True {
                              n179 = Multiply(x=w475, y="角度倍乘系数") -> (x*y=w474:dbl)
                            }
                          }
                        }
                        frame True {
                          n180 = Divide(x=w478, y=1.6) -> (x/y=w476:dbl)
                        }
                      }
                      n181 = local write "开光时间/ms"(w460) -> ()
                    }
                    frame True {
                      # "再次判断Δw，排除坏点影响"
                      n182 = local read "Δw2>C"() -> (w482:bool)
                      n183 = case shown="假" w482 {
                        tunnel: w483 -> [w488 _]
                        frame False {
                          n184 = local read "C=w-w0"() -> (w485:dbl)
                          n185 = local read "w0"() -> (w489:dbl)
                          n186 = Subtract(x=w489, y=w488) -> (x-y=w491:dbl)
                          n187 = Absolute Value(x=w491) -> (abs(x)=w490:dbl)
                          n188 = Add(x=w485, y=0.5) -> (x+y=w484:dbl)
                          n189 = Greater Or Equal?(x=w490, y=w484) -> (x >= y?=w487:bool)
                          n190 = case shown="真" w487 {
                            frame False {
                              n191 = local write "θi"(0.0 ("θi")) -> ()
                              n192 = local write "Δw1>C"(FALSE ("Δw1>C")) -> ()
                            }
                            frame True {
                              "Δw2>C" <- TRUE
                            }
                          }
                        }
                        frame True {
                        }
                      }
                    }
                  }
                  n193 = local read "Δw1>C"() -> (w439:bool)
                  n194 = local read "Δw2>C"() -> (w440:bool)
                  n195 = And(x=w439, y=w440) -> (x .and. y?=w438:bool)
                  n196 = case shown="真" w438 {
                    tunnel: w442 -> [_ w445]
                    frame False {
                    }
                    frame True {
                      # "4°后重置指示灯状态"
                      n197 = local read "θi"() -> (w449:dbl)
                      n198 = Subtract(x=w445, y=w449) -> (x-y=w450:dbl)
                      n199 = Absolute Value(x=w450) -> (abs(x)=w448:dbl)
                      n200 = Greater?(x=w448, y=4.0) -> (0:w446:bool)
                      n201 = case shown="真" w446 {
                        frame False {
                        }
                        frame True {
                          w451 = FALSE ("Δw1>C")
                          n202 = local write "Δw1>C"(w451) -> ()
                          n203 = local write "Δw2>C"(w451) -> ()
                          n204 = local write "θi"(0.0 ("θ")) -> ()
                        }
                      }
                    }
                  }
                }
              }
            }
            frame #11 {
              n205 = case shown="真" "是否移动光斑" {
                tunnel: w505 -> [w511 w522]
                tunnel: w504 -> [w510 w521]
                tunnel: [w511 w520] -> w503
                tunnel: [w510 w519] -> w502
                tunnel: w501 -> [w507 w518]
                tunnel: w500 -> [w508 w517]
                tunnel: w499 -> [w509 w516]
                tunnel: w498 -> [_ w515]
                tunnel: [w507 w514] -> w497
                tunnel: [w508 w513] -> w496
                tunnel: [w509 w512] -> w495
                frame False {
                }
                frame True {
                  n206 = stacked-sequence {
                    seq-local: [_ _ _ w664 _ _ _] -> [_ _ _ _ _ w761 _]
                    seq-local: [_ _ _ w661 _ _ _] -> [_ _ _ _ _ w760 _]
                    seq-local: [_ w537 _ _ _ _ _] -> [_ _ _ _ _ w764 _]
                    seq-local: [w524 _ _ _ _ _ _] -> [_ _ w652 _ _ _ _]
                    seq-local: [w523 _ _ _ _ _ _] -> [_ _ w651 _ _ _ _]
                    seq-local: [_ _ w649 _ _ _ _] -> [_ _ _ _ w747 _ _]
                    seq-local: [_ _ w650 _ _ _ _] -> [_ _ _ _ w748 _ _]
                    seq-local: [_ _ _ _ w746 _ _] -> [_ _ _ _ _ _ w839]
                    seq-local: [_ _ _ _ w745 _ _] -> [_ _ _ _ _ _ w838]
                    seq-local: [_ w538 _ _ _ _ _] -> [_ _ _ _ _ w765 _]
                    seq-local: [_ w536 _ _ _ _ _] -> [_ _ _ _ _ w763 _]
                    seq-local: [_ w535 _ _ _ _ _] -> [_ _ _ _ _ w762 _]
                    tunnel: w522 -> [w526 _ _ _ _ _ _]
                    tunnel: w521 -> [w525 _ _ _ _ _ _]
                    tunnel: [_ _ _ _ _ _ w841] -> w520
                    tunnel: [_ _ _ _ _ _ w840] -> w519
                    tunnel: w518 -> [_ w542 _ _ _ _ _]
                    tunnel: w517 -> [_ w541 _ _ _ _ _]
                    tunnel: w516 -> [_ w540 _ _ _ _ _]
                    tunnel: w515 -> [_ w539 _ _ _ _ _]
                    tunnel: [_ _ _ _ _ w759 _] -> w514
                    tunnel: [_ _ _ _ _ w758 _] -> w513
                    tunnel: [_ _ _ _ _ w757 _] -> w512
                    frame #0 {
                      # "开驱动光"
                      n207 = flat-sequence {
                        tunnel: [w530] -> w524
                        tunnel: [w529] -> w523
                        tunnel: w526 -> [w534]
                        tunnel: w525 -> [w533]
                        frame #0 {
                          n208 = local read "channel输出口"() -> (w528:i32)
                          n209 = Pick Line(multi-line string=":OUTP1 ON\n:OUTP2 ON" ("write buffer"), line index=w528) -> (output string=w531:string)  [unwired: 1 in]
                          n210 = local write "Output"(TRUE ("布尔")) -> ()
                          n211 = VISA Write(VISA resource name=w534, write buffer=w531, error in (no error)=w533) -> (VISA resource name out=w530:refnum<visa-resource-name>, error out=w529:errorcluster)  [unwired: 1 out]
                        }
                      }
                    }
                    frame #1 {
                      n212 = stacked-sequence {
                        seq-local: [w548 _ _ _] -> [_ w590 _ _]
                        seq-local: [w547 _ _ _] -> [_ w589 _ _]
                        seq-local: [w546 _ _ _] -> [_ _ _ _]
                        seq-local: [w545 _ _ _] -> [_ w588 _ _]
                        seq-local: [_ w571 _ _] -> [_ _ w604 _]
                        seq-local: [_ w570 _ _] -> [_ _ w603 _]
                        seq-local: [_ w569 _ _] -> [_ _ w602 _]
                        seq-local: [_ w568 _ _] -> [_ _ w601 _]
                        seq-local: [w544 _ _ _] -> [_ _ w607 _]
                        seq-local: [w543 _ _ _] -> [_ _ _ w620]
                        seq-local: [_ _ w594 _] -> [_ _ _ w628]
                        seq-local: [_ _ w593 _] -> [_ _ _ w627]
                        seq-local: [_ _ w592 _] -> [_ _ _ w626]
                        seq-local: [_ _ w591 _] -> [_ _ _ w625]
                        tunnel: w542 -> [w567 _ _ _]
                        tunnel: w541 -> [w566 _ _ _]
                        tunnel: w540 -> [w565 _ _ _]
                        tunnel: w539 -> [w564 _ _ _]
                        tunnel: [_ _ _ w624] -> w538
                        tunnel: [_ _ _ w623] -> w537
                        tunnel: [_ _ _ w622] -> w536
                        tunnel: [_ _ _ w621] -> w535
                        frame #0 {
                          w550 = 2 ("Motor")
                          w559 = 1 ("Motor")
                          w558 = 1 ("Setting")
                          # "设置闭环 获得当前位置"
                          n213 = call "SetCLEnabledSetting.vi"("CmdLib In"=w567, "DeviceKey In"=w566, "Device Address In"=w564, "Motor"=w559, "Setting"=w558, "error in (no error)"=w565) -> ("CmdLib Out"=w563:refnum<k24>, "DeviceKey Out"=w562:string, "Device Address Out"=w560:i32, "error out"=w561:errorcluster)  [unwired: 10 in]
                          n214 = call "GetPosition.vi"("CmdLib In"=w563, "DeviceKey In"=w562, "Device Address In"=w560, "Motor"=w559, "error in (no error)"=w561) -> ("CmdLib Out"=w554:refnum<k24>, "DeviceKey Out"=w555:string, "Device Address Out"=w556:i32, "Position"=w544:i32, "error out"=w557:errorcluster)  [unwired: 6 in]
                          "x" <- w544
                          n215 = call "SetCLEnabledSetting.vi"("CmdLib In"=w554, "DeviceKey In"=w555, "Device Address In"=w556, "Motor"=w550, "Setting"=w558, "error in (no error)"=w557) -> ("CmdLib Out"=w553:refnum<k24>, "DeviceKey Out"=w552:string, "Device Address Out"=w551:i32, "error out"=w549:errorcluster)  [unwired: 10 in]
                          n216 = call "GetPosition.vi"("CmdLib In"=w553, "DeviceKey In"=w552, "Device Address In"=w551, "Motor"=w550, "error in (no error)"=w549) -> ("CmdLib Out"=w548:refnum<k24>, "DeviceKey Out"=w547:string, "Device Address Out"=w545:i32, "Position"=w543:i32, "error out"=w546:errorcluster)  [unwired: 6 in]
                          "y" <- w543
                        }
                        frame #1 {
                          w575 = 2
                          w586 = 1
                          n217 = call "SetVelocity.vi"("CmdLib In"=w590, "DeviceKey In"=w589, "Device Address In"=w588, "Motor"=w586, "Steps Per Sec"="运动速度（步数/s）") -> ("CmdLib Out"=w583:refnum<k24>, "DeviceKey Out"=w584:string, "Device Address Out"=w587:i32, "error out"=w585:errorcluster)  [unwired: 11 in]
                          n218 = call "SetAcceleration.vi"("CmdLib In"=w583, "DeviceKey In"=w584, "Device Address In"=w587, "Motor"=w586, "Steps Per Sec 2"="运动加速度", "error in (no error)"=w585) -> ("CmdLib Out"=w582:refnum<k24>, "DeviceKey Out"=w581:string, "Device Address Out"=w580:i32, "error out"=w578:errorcluster)  [unwired: 10 in]
                          n219 = call "SetVelocity.vi"("CmdLib In"=w582, "DeviceKey In"=w581, "Device Address In"=w580, "Motor"=w575, "Steps Per Sec"="运动速度（步数/s）", "error in (no error)"=w578) -> ("CmdLib Out"=w576:refnum<k24>, "DeviceKey Out"=w572:string, "Device Address Out"=w573:i32, "error out"=w577:errorcluster)  [unwired: 10 in]
                          n220 = call "SetAcceleration.vi"("CmdLib In"=w576, "DeviceKey In"=w572, "Device Address In"=w573, "Motor"=w575, "Steps Per Sec 2"="运动加速度", "error in (no error)"=w577) -> ("CmdLib Out"=w571:refnum<k24>, "DeviceKey Out"=w570:string, "Device Address Out"=w569:i32, "error out"=w568:errorcluster)  [unwired: 10 in]
                        }
                        frame #2 {
                          w595 = 1 ("Motor")
                          n221 = Multiply(x="x初次移动/um", y="x比例(步/um)") -> (x*y=w605:dbl)
                          n222 = Round To Nearest(number=w605) -> (nearest integer value=w606:dbl)
                          n223 = Add(x=w607, y=w606) -> (x+y=w600:dbl)
                          n224 = call "AbsoluteMove.vi"("CmdLib In"=w604, "DeviceKey In"=w603, "Device Address In"=w602, "Motor"=w595, "Target Pos"=w600, "error in (no error)"=w601) -> ("CmdLib Out"=w599:refnum<k24>, "DeviceKey Out"=w598:string, "Device Address Out"=w597:i32, "error out"=w596:errorcluster)  [unwired: 10 in]
                          n225 = while {
                            tunnel: w599 -> [w619]
                            tunnel: w598 -> [w618]
                            tunnel: w597 -> [w617]
                            tunnel: w595 -> [w615]
                            shift-right: [w613] -> w591
                            shift-left: w596 -> [w616]
                            tunnel: [w612] -> w594
                            tunnel: [w611] -> w593
                            tunnel: [w610] -> w592
                            stop <- w614 stop-if-true
                            n226 = call "GetMotionDone.vi"("CmdLib In"=w619, "DeviceKey In"=w618, "Device Address In"=w617, "Motor"=w615, "error in (no error)"=w616) -> ("CmdLib Out"=w612:refnum<k24>, "DeviceKey Out"=w611:string, "Device Address Out"=w610:i32, "Is Motion Done"=w614:bool, "error out"=w613:errorcluster)  [unwired: 6 in]
                          }
                        }
                        frame #3 {
                          w629 = 2 ("Motor")
                          n227 = Multiply(x="y初次移动/um", y="y比例(步/um)") -> (x*y=w635:dbl)
                          n228 = Round To Nearest(number=w635) -> (nearest integer value=w636:dbl)
                          n229 = Add(x=w620, y=w636) -> (x+y=w634:dbl)
                          n230 = call "AbsoluteMove.vi"("CmdLib In"=w628, "DeviceKey In"=w627, "Device Address In"=w626, "Motor"=w629, "Target Pos"=w634, "error in (no error)"=w625) -> ("CmdLib Out"=w633:refnum<k24>, "DeviceKey Out"=w632:string, "Device Address Out"=w631:i32, "error out"=w630:errorcluster)  [unwired: 10 in]
                          n231 = while {
                            tunnel: w633 -> [w648]
                            tunnel: w632 -> [w647]
                            tunnel: w631 -> [w646]
                            tunnel: w629 -> [w644]
                            shift-right: [w642] -> w621
                            shift-left: w630 -> [w645]
                            tunnel: [w641] -> w624
                            tunnel: [w640] -> w623
                            tunnel: [w639] -> w622
                            stop <- w643 stop-if-true
                            n232 = call "GetMotionDone.vi"("CmdLib In"=w648, "DeviceKey In"=w647, "Device Address In"=w646, "Motor"=w644, "error in (no error)"=w645) -> ("CmdLib Out"=w641:refnum<k24>, "DeviceKey Out"=w640:string, "Device Address Out"=w639:i32, "Is Motion Done"=w643:bool, "error out"=w642:errorcluster)  [unwired: 6 in]
                          }
                        }
                      }
                    }
                    frame #2 {
                      n233 = flat-sequence {
                        tunnel: w652 -> [w660]
                        tunnel: w651 -> [w659]
                        tunnel: [w656] -> w650
                        tunnel: [w655] -> w649
                        frame #0 {
                          n234 = local read "channel输出口"() -> (w654:i32)
                          n235 = Pick Line(multi-line string=":OUTP1 OFF\n:OUTP2 OFF" ("write buffer"), line index=w654) -> (output string=w657:string)  [unwired: 1 in]
                          n236 = local write "Output"(FALSE ("布尔")) -> ()
                          n237 = VISA Write(VISA resource name=w660, write buffer=w657, error in (no error)=w659) -> (VISA resource name out=w656:refnum<visa-resource-name>, error out=w655:errorcluster)  [unwired: 1 out]
                        }
                      }
                    }
                    frame #3 {
                      # "识别两个位置"
                      n238 = Multiply(x="截图等待时间（秒）", y=u32 1000) -> (x*y=w667:u32)
                      n239 = Wait (ms)(milliseconds to wait=w667) -> ()  [unwired: 1 out]
                      n240 = stacked-sequence {
                        seq-local: [w684 _ _ _ _ _] -> [_ w697 w706 w716 w726 w736]
                        tunnel: [_ _ _ w715 _ _] -> w672
                        tunnel: [_ _ w705 _ _ _] -> w673
                        tunnel: [_ _ _ _ w725 _] -> w671
                        tunnel: [_ _ _ _ _ w735] -> w670
                        frame #0 {
                          n241 = Get Date/Time In Seconds() -> (seconds since 1Jan1904=w693:timestamp)
                          n242 = Get Date/Time String(date format (0)=enum16{"short", "long", "abbreviated"}."abbreviated" ("日期格式(0)"), seconds (now)=w693, want seconds? (F)=TRUE ("需要秒？(F)")) -> (date string=w696:string, time string=w694:string)
                          n243 = Search and Replace String(replace all?=TRUE ("替换全部？(F)"), input string=w694, search string=":" ("搜索字符串"), replace string="-" ("替换字符串(\"\")")) -> (result string=w695:string)  [unwired: 4 in, 3 out]
                          n244 = Concatenate Strings("D:\\desktop\\train\\photo\\", w696, w695, "光谱" ("字符串"), ".jpg" ("字符串")) -> (w684:string)
                        }
                        frame #1 {
                          n245 = Open Python Session(python version="3.9" ("Python version")) -> (session out=w704:refnum<k35>, error out=w702:errorcluster)  [unwired: 2 in]
                          n246 = node(w704, path "D:/desktop/train/model/main.py" ("module path"), "screenshot" ("function name"), w702, w697) -> (w703:refnum<k35>, w701:errorcluster)  [unwired: 3 in, 2 out]
                          n247 = Close Python Session(session in=w703, error in=w701) -> ()  [unwired: 1 out]
                        }
                        frame #2 {
                          n248 = Open Python Session(python version="3.9" ("Python version")) -> (session out=w713:refnum<k35>, error out=w711:errorcluster)  [unwired: 2 in]
                          n249 = node(w713, path "D:/desktop/train/newpro.py" ("module path"), "funx" ("function name"), w711, 0.0, w706) -> (w712:refnum<k35>, w710:errorcluster, w705:dbl)  [unwired: 1 in, 2 out]
                          n250 = Close Python Session(session in=w712, error in=w710) -> ()  [unwired: 1 out]
                        }
                        frame #3 {
                          n251 = Open Python Session(python version="3.9" ("Python version")) -> (session out=w723:refnum<k35>, error out=w721:errorcluster)  [unwired: 2 in]
                          n252 = node(w723, path "D:/desktop/train/newpro.py" ("module path"), "funy" ("function name"), w721, 0.0, w716) -> (w722:refnum<k35>, w717:errorcluster, w715:dbl)  [unwired: 1 in, 2 out]
                          n253 = Close Python Session(session in=w722, error in=w717) -> ()  [unwired: 1 out]
                        }
                        frame #4 {
                          n254 = Open Python Session(python version="3.9" ("Python version")) -> (session out=w733:refnum<k35>, error out=w731:errorcluster)  [unwired: 2 in]
                          n255 = node(w733, path "D:/desktop/train/newpro_wan.py" ("module path"), "funx" ("function name"), w731, 0.0, w726) -> (w732:refnum<k35>, w730:errorcluster, w725:dbl)  [unwired: 1 in, 2 out]
                          n256 = Close Python Session(session in=w732, error in=w730) -> ()  [unwired: 1 out]
                        }
                        frame #5 {
                          n257 = Open Python Session(python version="3.9" ("Python version")) -> (session out=w743:refnum<k35>, error out=w741:errorcluster)  [unwired: 2 in]
                          n258 = node(w743, path "D:/desktop/train/newpro_wan.py" ("module path"), "funy" ("function name"), w741, 0.0, w736) -> (w742:refnum<k35>, w740:errorcluster, w735:dbl)  [unwired: 1 in, 2 out]
                          n259 = Close Python Session(session in=w742, error in=w740) -> ()  [unwired: 1 out]
                        }
                      }
                      n260 = Subtract(x=w672, y=w670) -> (x-y=w674:dbl)
                      n261 = case shown="假" "y是否取反" {
                        tunnel: w674 -> [w678 w680]
                        tunnel: [w678 w679] -> w662
                        frame False {
                        }
                        frame True {
                          n262 = Negate(x=w680) -> (-x=w679:dbl)
                        }
                      }
                      n263 = Subtract(x=w673, y=w671) -> (x-y=w675:dbl)
                      n264 = case shown="假" "x是否取反" {
                        tunnel: w675 -> [w681 w683]
                        tunnel: [w681 w682] -> w665
                        frame False {
                        }
                        frame True {
                          n265 = Negate(x=w683) -> (-x=w682:dbl)
                        }
                      }
                      n266 = local read "画面长度（um）"() -> (w663:dbl)
                      n267 = Multiply(x=w665, y="画面长度（um）") -> (x*y=w664:dbl)
                      n268 = Multiply(x=w662, y=w663) -> (x*y=w661:dbl)
                    }
                    frame #4 {
                      n269 = flat-sequence {
                        tunnel: w748 -> [w756]
                        tunnel: w747 -> [w755]
                        tunnel: [w752] -> w746
                        tunnel: [w751] -> w745
                        frame #0 {
                          n270 = local read "channel输出口"() -> (w750:i32)
                          n271 = Pick Line(multi-line string=":OUTP1 ON\n:OUTP2 ON" ("write buffer"), line index=w750) -> (output string=w753:string)  [unwired: 1 in]
                          n272 = local write "Output"(TRUE ("布尔")) -> ()
                          n273 = VISA Write(VISA resource name=w756, write buffer=w753, error in (no error)=w755) -> (VISA resource name out=w752:refnum<visa-resource-name>, error out=w751:errorcluster)  [unwired: 1 out]
                        }
                      }
                    }
                    frame #5 {
                      # "移动光斑"
                      n274 = stacked-sequence {
                        seq-local: [w779 _ _] -> [_ _ _]
                        seq-local: [w778 _ _] -> [_ _ _]
                        seq-local: [w777 _ _] -> [_ _ _]
                        seq-local: [w776 _ _] -> [_ _ _]
                        seq-local: [w771 _ _] -> [_ w798 _]
                        seq-local: [w770 _ _] -> [_ _ w814]
                        seq-local: [_ w790 _] -> [_ _ w821]
                        seq-local: [_ w789 _] -> [_ _ w820]
                        seq-local: [_ w788 _] -> [_ _ w819]
                        seq-local: [_ w787 _] -> [_ _ w818]
                        tunnel: [_ _ w817] -> w759
                        tunnel: [_ _ w816] -> w758
                        tunnel: [_ _ w815] -> w757
                        tunnel: w765 -> [w775 _ _]
                        tunnel: w764 -> [w774 _ _]
                        tunnel: w763 -> [w773 _ _]
                        tunnel: w762 -> [w772 _ _]
                        tunnel: w761 -> [_ w786 _]
                        tunnel: w760 -> [_ _ w813]
                        frame #0 {
                          # "获得当前位置"
                          n275 = call "GetPosition.vi"("CmdLib In"=w775, "DeviceKey In"=w774, "Device Address In"=w773, "Motor"=1, "error in (no error)"=w772) -> ("CmdLib Out"=w769:refnum<k24>, "DeviceKey Out"=w768:string, "Device Address Out"=w767:i32, "Position"=w771:i32, "error out"=w766:errorcluster)  [unwired: 6 in]
                          n276 = local write "x"(w771) -> ()
                          n277 = call "GetPosition.vi"("CmdLib In"=w769, "DeviceKey In"=w768, "Device Address In"=w767, "Motor"=2, "error in (no error)"=w766) -> ("CmdLib Out"=w779:refnum<k24>, "DeviceKey Out"=w778:string, "Device Address Out"=w776:i32, "Position"=w770:i32, "error out"=w777:errorcluster)  [unwired: 6 in]
                          n278 = local write "y"(w770) -> ()
                        }
                        frame #1 {
                          w791 = 1 ("Motor")
                          n279 = local read "x比例(步/um)"() -> (w785:dbl)
                          n280 = Multiply(x=w786, y=w785) -> (x*y=w783:dbl)
                          n281 = Multiply(x=w783, y="Δx系数（0-1之间）") -> (x*y=w782:dbl)
                          n282 = Round To Nearest(number=w782) -> (nearest integer value=w797:dbl)
                          n283 = Add(x=w798, y=w797) -> (x+y=w796:dbl)
                          n284 = call "AbsoluteMove.vi"("Motor"=w791, "Target Pos"=w796) -> ("CmdLib Out"=w795:refnum<k24>, "DeviceKey Out"=w794:string, "Device Address Out"=w793:i32, "error out"=w792:errorcluster)  [unwired: 14 in]
                          n285 = while {
                            tunnel: w795 -> [w808]
                            tunnel: w794 -> [w807]
                            tunnel: w793 -> [w806]
                            tunnel: w791 -> [w804]
                            shift-right: [w802] -> w787
                            shift-left: w792 -> [w805]
                            tunnel: [w801] -> w790
                            tunnel: [w800] -> w789
                            tunnel: [w799] -> w788
                            stop <- w803 stop-if-true
                            n286 = call "GetMotionDone.vi"("CmdLib In"=w808, "DeviceKey In"=w807, "Device Address In"=w806, "Motor"=w804, "error in (no error)"=w805) -> ("CmdLib Out"=w801:refnum<k24>, "DeviceKey Out"=w800:string, "Device Address Out"=w799:i32, "Is Motion Done"=w803:bool, "error out"=w802:errorcluster)  [unwired: 6 in]
                          }
                        }
                        frame #2 {
                          w822 = 2 ("Motor")
                          n287 = local read "y比例(步/um)"() -> (w812:dbl)
                          n288 = Multiply(x=w813, y=w812) -> (x*y=w810:dbl)
                          n289 = Multiply(x=w810, y="Δy系数（0-1之间）") -> (x*y=w809:dbl)
                          n290 = Round To Nearest(number=w809) -> (nearest integer value=w828:dbl)
                          n291 = Add(x=w814, y=w828) -> (x+y=w827:dbl)
                          n292 = call "AbsoluteMove.vi"("CmdLib In"=w821, "DeviceKey In"=w820, "Device Address In"=w819, "Motor"=w822, "Target Pos"=w827, "error in (no error)"=w818) -> ("CmdLib Out"=w826:refnum<k24>, "DeviceKey Out"=w825:string, "Device Address Out"=w824:i32, "error out"=w823:errorcluster)  [unwired: 10 in]
                          n293 = while {
                            tunnel: w826 -> [w837]
                            tunnel: w825 -> [w836]
                            tunnel: w824 -> [w835]
                            tunnel: w822 -> [w833]
                            shift-right: [w831] -> w815
                            shift-left: w823 -> [w834]
                            tunnel: [w830] -> w817
                            tunnel: [w829] -> w816
                            stop <- w832 stop-if-true
                            n294 = call "GetMotionDone.vi"("CmdLib In"=w837, "DeviceKey In"=w836, "Device Address In"=w835, "Motor"=w833, "error in (no error)"=w834) -> ("CmdLib Out"=w830:refnum<k24>, "DeviceKey Out"=w829:string, "Is Motion Done"=w832:bool, "error out"=w831:errorcluster)  [unwired: 6 in, 1 out]
                          }
                        }
                      }
                    }
                    frame #6 {
                      # "关驱动光"
                      n295 = flat-sequence {
                        tunnel: w839 -> [w849]
                        tunnel: w838 -> [w848]
                        tunnel: [w845] -> w841
                        tunnel: [w844] -> w840
                        frame #0 {
                          n296 = local read "channel输出口"() -> (w843:i32)
                          n297 = Pick Line(multi-line string=":OUTP1 OFF\n:OUTP2 OFF" ("write buffer"), line index=w843) -> (output string=w846:string)  [unwired: 1 in]
                          n298 = local write "Output"(FALSE ("布尔")) -> ()
                          n299 = VISA Write(VISA resource name=w849, write buffer=w846, error in (no error)=w848) -> (VISA resource name out=w845:refnum<visa-resource-name>, error out=w844:errorcluster)  [unwired: 1 out]
                        }
                      }
                    }
                  }
                }
              }
            }
            frame #12 {
              n300 = local write "正在测量"(FALSE) -> ()
            }
          }
          n301 = Build Array(w186, w185, w184, w183, w179) -> (w177:dbl[])
          n302 = local read "结果展示"() -> (w176:dbl[][])
          n303 = Insert Into Array(array=w176, new element=w177) -> (→"结果展示":dbl[][])  [unwired: 2 in]
        }
        n304 = VISA Close(VISA resource name=w137, error in (no error)=w136) -> (error out=→"output control error":errorcluster)
        n305 = VISA Close(VISA resource name=w140, error in (no error)=w139) -> (error out=→"照明光error out":errorcluster)
        n306 = Path To String(path=w113) -> (string=w122:string)
        n307 = local write "结果展示"(dbl[][] [] ("结果展示")) -> ()
        n308 = Concatenate Strings(w122, "循环汇总" ("字符串"), ".xls" ("字符串")) -> (w121:string)
        n309 = String To Path(string=w121) -> (path=w120:path)
        n310 = call-poly <vilib>:"Write Delimited Spreadsheet.vi"("file path (dialog if empty)"=w120, "format (%.3f)"="%.16f", "2D data"=w116, "append to file? (new file:F)"=TRUE ("append to file? (F)"), "transpose? (no:F)"=FALSE ("transpose? (F)")) -> ()  [unwired: 9 in, 2 out]
        n311 = call "DeviceClose.vi"("error in (no error)"=w99, "DeviceKey In"=w100, "CmdLib In"=w101) -> ("error out"=w97:errorcluster, "CmdLib Out"=w98:refnum<k24>)  [unwired: 2 in, 1 out]
        n312 = call "Shutdown.vi"("error in (no error)"=w97, "CmdLib In"=w98) -> ("error out"=→"error out 2":errorcluster)  [unwired: 4 in, 1 out]
      }
    }
    n313 = event shown="[1] \"低电平持续输出\": 值改变" {
      selector: _ -> [_ _]
      dyn-events: _ -> [_ _]
      timeout: u32 0 ("Time") -> [_ _]
      tunnel: "低电平持续输出" -> [_ w880]
      event Timeout {
        n314 = event-data() -> ()  [unwired: 1 in, 2 out]
      }
      event "低电平持续输出": Value Change {
        w884 = " :SOUR1\n :SOUR2"  # Channel
        n315 = event-data() -> ()  [unwired: 1 in, 6 out]
        n316 = local read "channel输出口"() -> (w885:i32)
        n317 = Pick Line(multi-line string=w884, line index=w885) -> (output string=w883:string)  [unwired: 1 in]
        n318 = local read "VISA 信号发生器"() -> (w888:refnum<visa-resource-name>)
        n319 = VISA Open(VISA resource name=w888) -> (VISA resource name=w887:refnum<visa-resource-name>, error out=w886:errorcluster)  [unwired: 4 in]
        n320 = stacked-sequence {
          seq-local: [w894 _ _ _ _ _ _ _ _ _ _ _ _] -> [_ _ w909 _ _ _ _ _ _ _ _ _ _]
          seq-local: [w893 _ _ _ _ _ _ _ _ _ _ _ _] -> [_ _ w908 _ _ _ _ _ _ _ _ _ _]
          seq-local: [_ _ w907 _ _ _ _ _ _ _ _ _ _] -> [_ _ _ _ w912 _ _ _ _ _ _ _ _]
          seq-local: [_ _ w906 _ _ _ _ _ _ _ _ _ _] -> [_ _ _ _ w913 _ _ _ _ _ _ _ _]
          seq-local: [_ _ _ _ w921 _ _ _ _ _ _ _ _] -> [_ _ _ _ _ _ w932 _ _ _ _ _ _]
          seq-local: [_ _ _ _ w920 _ _ _ _ _ _ _ _] -> [_ _ _ _ _ _ w931 _ _ _ _ _ _]
          seq-local: [_ _ _ _ _ _ w925 _ _ _ _ _ _] -> [_ _ _ _ _ _ _ _ w935 _ _ _ _]
          seq-local: [_ _ _ _ _ _ w924 _ _ _ _ _ _] -> [_ _ _ _ _ _ _ _ w934 _ _ _ _]
          seq-local: [_ _ _ _ _ _ _ _ w938 _ _ _ _] -> [_ _ _ _ _ _ _ _ _ _ w949 _ _]
          seq-local: [_ _ _ _ _ _ _ _ w937 _ _ _ _] -> [_ _ _ _ _ _ _ _ _ _ w948 _ _]
          seq-local: [_ _ _ _ _ _ _ _ _ _ w946 _ _] -> [_ _ _ _ _ _ _ _ _ _ _ _ w963]
          seq-local: [_ _ _ _ _ _ _ _ _ _ w945 _ _] -> [_ _ _ _ _ _ _ _ _ _ _ _ w962]
          tunnel: w887 -> [w899 _ _ _ _ _ _ _ _ _ _ _ _]
          tunnel: w886 -> [w892 _ _ _ _ _ _ _ _ _ _ _ _]
          tunnel: w883 -> [w891 _ w905 _ w918 _ w929 _ w939 _ w952 _ _]
          tunnel: [_ _ _ _ _ _ _ _ _ _ _ _ w961] -> w882
          tunnel: [_ _ _ _ _ _ _ _ _ _ _ _ w959] -> w881
          tunnel: w880 -> [_ _ _ _ _ _ _ _ _ _ _ _ w960]
          frame #0 {
            w896 = " PULSe"  # Function Command
            n321 = local read "输出信号波形"() -> (w890:u16)
            n322 = Concatenate Strings(w891, ":FUNC" ("string (\"\")")) -> (w897:string)
            n323 = Pick Line(string ("")=w897, multi-line string=w896, line index=w890) -> (output string=w895:string)
            n324 = VISA Write(VISA resource name=w899, write buffer=w895, error in (no error)=w892) -> (VISA resource name out=w894:refnum<visa-resource-name>, error out=w893:errorcluster)  [unwired: 1 out]
          }
          frame #1 {
            n325 = Wait (ms)(milliseconds to wait=u32 150) -> ()  [unwired: 1 out]
          }
          frame #2 {
            n326 = Number To Fractional String(use system decimal point (T)=TRUE ("使用系统小数点(T)"), number=1.0 ("数字")) -> (F-format string=w903:string)  [unwired: 2 in]
            n327 = Concatenate Strings ("连接字符串")(w905, ":VOLTage：HIGH ", w903) -> (w902:string)
            n328 = VISA Write(VISA resource name=w909, write buffer=w902, error in (no error)=w908) -> (VISA resource name out=w907:refnum<visa-resource-name>, error out=w906:errorcluster)  [unwired: 1 out]
          }
          frame #3 {
            n329 = Wait (ms)(milliseconds to wait=u32 150) -> ()  [unwired: 1 out]
          }
          frame #4 {
            # "1 电压偏置"
            n330 = Number To Fractional String(use system decimal point (T)=TRUE ("使用系统小数点(T)"), number=0.0 ("数字")) -> (F-format string=w916:string)  [unwired: 2 in]
            n331 = Concatenate Strings(w918, ":VOLTage:LOW ", w916) -> (w917:string)
            n332 = VISA Write(VISA resource name=w912, write buffer=w917, error in (no error)=w913) -> (VISA resource name out=w921:refnum<visa-resource-name>, error out=w920:errorcluster)  [unwired: 1 out]
          }
          frame #5 {
            n333 = Wait (ms)(milliseconds to wait=u32 150) -> ()  [unwired: 1 out]
          }
          frame #6 {
            n334 = local read "channel输出口"() -> (w927:i32)
            n335 = Pick Line(multi-line string=":OUTP1:IMPedance \n:OUTP2:IMPedance " ("write buffer"), line index=w927) -> (output string=w926:string)  [unwired: 1 in]
            n336 = Concatenate Strings ("连接字符串")(w929, w926, "INFINITY") -> (w930:string)
            n337 = VISA Write(VISA resource name=w932, write buffer=w930, error in (no error)=w931) -> (VISA resource name out=w925:refnum<visa-resource-name>, error out=w924:errorcluster)  [unwired: 1 out]
          }
          frame #7 {
            n338 = Wait (ms)(milliseconds to wait=u32 150) -> ()  [unwired: 1 out]
          }
          frame #8 {
            n339 = Number To Fractional String(use system decimal point (T)=TRUE ("使用系统小数点(T)"), number=0.0 ("数字")) -> (F-format string=w942:string)  [unwired: 2 in]
            n340 = Concatenate Strings(w939, ":PULSe:DELay ", w942) -> (w940:string)
            n341 = VISA Write(VISA resource name=w935, write buffer=w940, error in (no error)=w934) -> (VISA resource name out=w938:refnum<visa-resource-name>, error out=w937:errorcluster)  [unwired: 1 out]
          }
          frame #9 {
            n342 = Wait (ms)(milliseconds to wait=u32 150) -> ()  [unwired: 1 out]
          }
          frame #10 {
            w953 = ":LEADing\n:TRAiling "  # Channel
            w957 = ":PULSe:TRANsition"  # VOLTage:Offset
            n343 = local read "上升下降沿"() -> (w954:i32)
            n344 = Pick Line(multi-line string=w953, line index=w954) -> (output string=w950:string)  [unwired: 1 in]
            n345 = Number To Fractional String(use system decimal point (T)=TRUE ("使用系统小数点(T)"), number=0.0 ("数字")) -> (F-format string=w951:string)  [unwired: 2 in]
            n346 = Concatenate Strings(w952, w957, w950, w951) -> (w955:string)
            n347 = VISA Write(VISA resource name=w949, write buffer=w955, error in (no error)=w948) -> (VISA resource name out=w946:refnum<visa-resource-name>, error out=w945:errorcluster)  [unwired: 1 out]
          }
          frame #11 {
            n348 = Wait (ms)(milliseconds to wait=u32 150) -> ()  [unwired: 1 out]
          }
          frame #12 {
            n349 = case shown="假" w960 {
              tunnel: w963 -> [w971 w972]
              tunnel: [w970 w979] -> w959
              tunnel: w962 -> [w969 w977]
              tunnel: [w968 w978] -> w961
              frame True {
                n350 = local write "Output"(TRUE ("布尔")) -> ()
                n351 = local read "channel输出口"() -> (w965:i32)
                n352 = Pick Line(multi-line string=":OUTP1 ON\n:OUTP2 ON" ("write buffer"), line index=w965) -> (output string=w964:string)  [unwired: 1 in]
                n353 = VISA Write(VISA resource name=w971, write buffer=w964, error in (no error)=w969) -> (VISA resource name out=w968:refnum<visa-resource-name>, error out=w970:errorcluster)  [unwired: 1 out]
              }
              frame False {
                n354 = local read "channel输出口"() -> (w974:i32)
                n355 = Pick Line(multi-line string=":OUTP1 OFF\n:OUTP2 OFF" ("write buffer"), line index=w974) -> (output string=w973:string)  [unwired: 1 in]
                n356 = VISA Write(VISA resource name=w972, write buffer=w973, error in (no error)=w977) -> (VISA resource name out=w978:refnum<visa-resource-name>, error out=w979:errorcluster)  [unwired: 1 out]
                n357 = local write "Output"(FALSE ("布尔")) -> ()
              }
            }
          }
        }
        n358 = VISA Close(VISA resource name=w882, error in (no error)=w881) -> (error out=→"output control error  4":errorcluster)
      }
    }
    n359 = event shown="[1] \"Enable\": 值改变" {
      selector: _ -> [_ _]
      dyn-events: _ -> [_ _]
      timeout: u32 0 ("Time") -> [_ _]
      tunnel: "Enable" -> [_ w855]
      event Timeout {
        n360 = event-data() -> ()  [unwired: 1 in, 2 out]
      }
      event "Enable": Value Change {
        n361 = event-data() -> ()  [unwired: 1 in, 6 out]
        n362 = local read "VISA 信号发生器"() -> (w851:refnum<visa-resource-name>)
        n363 = VISA Open(VISA resource name=w851) -> (VISA resource name=w854:refnum<visa-resource-name>, error out=w857:errorcluster)  [unwired: 4 in]
        n364 = stacked-sequence {
          tunnel: w855 -> [w862 _]
          tunnel: w857 -> [w861 _]
          tunnel: w854 -> [w860 _]
          tunnel: [w859 _] -> w853
          tunnel: [w858 _] -> w852
          frame #0 {
            n365 = case shown="真" w862 {
              tunnel: w860 -> [w870 w878]
              tunnel: [w869 w877] -> w858
              tunnel: w861 -> [w868 w875]
              tunnel: [w867 w876] -> w859
              frame True {
                n366 = local write "Output"(TRUE ("布尔")) -> ()
                n367 = local read "channel输出口"() -> (w864:i32)
                n368 = Pick Line(multi-line string=":OUTP1 ON\n:OUTP2 ON" ("write buffer"), line index=w864) -> (output string=w863:string)  [unwired: 1 in]
                n369 = VISA Write(VISA resource name=w870, write buffer=w863, error in (no error)=w868) -> (VISA resource name out=w867:refnum<visa-resource-name>, error out=w869:errorcluster)  [unwired: 1 out]
              }
              frame False {
                n370 = local read "channel输出口"() -> (w872:i32)
                n371 = Pick Line(multi-line string=":OUTP1 OFF\n:OUTP2 OFF" ("write buffer"), line index=w872) -> (output string=w871:string)  [unwired: 1 in]
                n372 = VISA Write(VISA resource name=w878, write buffer=w871, error in (no error)=w875) -> (VISA resource name out=w876:refnum<visa-resource-name>, error out=w877:errorcluster)  [unwired: 1 out]
                n373 = local write "Output"(FALSE ("布尔")) -> ()
              }
            }
          }
          frame #1 {
            n374 = Wait (ms)(milliseconds to wait=u32 150) -> ()  [unwired: 1 out]
          }
        }
        n375 = VISA Close(VISA resource name=w853, error in (no error)=w852) -> (error out=→"output control error  5":errorcluster)
      }
    }
    n376 = event shown="[1] \"Enable 2\": 值改变" {
      selector: _ -> [_ _]
      dyn-events: _ -> [_ _]
      timeout: u32 0 ("Time") -> [_ _]
      tunnel: "Enable 2" -> [_ w27]
      event Timeout {
        n377 = event-data() -> ()  [unwired: 1 in, 2 out]
      }
      event "Enable 2": Value Change {
        n378 = event-data() -> ()  [unwired: 1 in, 6 out]
        n379 = Not(x=w27) -> (.not. x?=w26:bool)
        n380 = local read "VISA 信号发生器"() -> (w28:refnum<visa-resource-name>)
        n381 = VISA Open(VISA resource name=w28) -> (VISA resource name=w31:refnum<visa-resource-name>, error out=w32:errorcluster)  [unwired: 4 in]
        n382 = stacked-sequence {
          tunnel: w26 -> [w37 _]
          tunnel: w32 -> [w36 _]
          tunnel: w31 -> [w35 _]
          tunnel: [w34 _] -> w30
          tunnel: [w33 _] -> w29
          frame #0 {
            n383 = case shown="真" w37 {
              tunnel: w35 -> [w46 w57]
              tunnel: [w45 w56] -> w33
              tunnel: w36 -> [w44 w54]
              tunnel: [w43 w55] -> w34
              frame True {
                n384 = local read "channel输出口"() -> (w39:i32)
                n385 = local write "Output 2"(FALSE ("布尔")) -> ()
                n386 = case shown="1" w39 {
                  tunnel: [1 0] -> w38
                  frame 0, Default {
                  }
                  frame 1 {
                  }
                }
                n387 = Pick Line(multi-line string=":OUTP1 ON\n:OUTP2 ON" ("write buffer"), line index=w38) -> (output string=w40:string)  [unwired: 1 in]
                n388 = VISA Write(VISA resource name=w46, write buffer=w40, error in (no error)=w44) -> (VISA resource name out=w43:refnum<visa-resource-name>, error out=w45:errorcluster)  [unwired: 1 out]
              }
              frame False {
                n389 = local read "channel输出口"() -> (w50:i32)
                n390 = case shown="1" w50 {
                  tunnel: [1 0] -> w49
                  frame 0, Default {
                  }
                  frame 1 {
                  }
                }
                n391 = Pick Line(multi-line string=":OUTP1 OFF\n:OUTP2 OFF" ("write buffer"), line index=w49) -> (output string=w51:string)  [unwired: 1 in]
                n392 = VISA Write(VISA resource name=w57, write buffer=w51, error in (no error)=w54) -> (VISA resource name out=w55:refnum<visa-resource-name>, error out=w56:errorcluster)  [unwired: 1 out]
                n393 = local write "Output 2"(TRUE ("布尔")) -> ()
              }
            }
          }
          frame #1 {
            n394 = Wait (ms)(milliseconds to wait=u32 150) -> ()  [unwired: 1 out]
          }
        }
        n395 = VISA Close(VISA resource name=w30, error in (no error)=w29) -> ()  [unwired: 1 out]
      }
    }
    n396 = case shown="真" "设置参数" {
      frame False {
      }
      frame True {
        w986 = " :SOUR1\n :SOUR2"  # Channel
        n397 = local read "VISA 信号发生器"() -> (w988:refnum<visa-resource-name>)
        n398 = local read "channel输出口"() -> (w987:i32)
        n399 = case shown="1" w987 {
          tunnel: [1 0] -> w980
          frame 0, Default {
          }
          frame 1 {
          }
        }
        n400 = VISA Open(VISA resource name=w988) -> (VISA resource name=w991:refnum<visa-resource-name>, error out=w992:errorcluster)  [unwired: 4 in]
        n401 = Pick Line(multi-line string=w986, line index=w980) -> (output string=w981:string)  [unwired: 1 in]
        n402 = Pick Line(multi-line string=w986, line index=w987) -> (output string=w989:string)  [unwired: 1 in]
        n403 = stacked-sequence {
          seq-local: [w1088 _ _ _ _ _ _ _ _ _ _ _ _ _ _] -> [_ _ w1103 _ _ _ _ _ _ _ _ _ _ _ _]
          seq-local: [w1087 _ _ _ _ _ _ _ _ _ _ _ _ _ _] -> [_ _ w1102 _ _ _ _ _ _ _ w1141 _ _ _ _]
          seq-local: [_ _ w1101 _ _ _ _ _ _ _ _ _ _ _ _] -> [_ _ _ _ w1112 _ _ _ _ _ _ _ _ _ _]
          seq-local: [_ _ w1100 _ _ _ _ _ _ _ _ _ _ _ _] -> [_ _ _ _ w1111 _ _ _ _ _ _ _ _ _ _]
          seq-local: [_ _ _ _ w1110 _ _ _ _ _ _ _ _ _ _] -> [_ _ _ _ _ _ w1118 _ _ _ _ _ _ _ _]
          seq-local: [_ _ _ _ w1107 _ _ _ _ _ _ _ _ _ _] -> [_ _ _ _ _ _ w1117 _ _ _ _ _ _ _ _]
          seq-local: [_ _ _ _ _ _ w1125 _ _ _ _ _ _ _ _] -> [_ _ _ _ _ _ _ _ w1136 _ _ _ _ _ _]
          seq-local: [_ _ _ _ _ _ w1124 _ _ _ _ _ _ _ _] -> [_ _ _ _ _ _ _ _ w1135 _ _ _ _ _ _]
          seq-local: [_ _ _ _ _ _ _ _ w1129 _ _ _ _ _ _] -> [_ _ _ _ _ _ _ _ _ _ w1142 _ _ _ _]
          seq-local: [_ _ _ _ _ _ _ _ w1128 _ _ _ _ _ _] -> [_ _ _ _ _ _ _ _ _ _ _ _ _ _ _]
          seq-local: [_ _ _ _ _ _ _ _ _ _ w1138 _ _ _ _] -> [_ _ _ _ _ _ _ _ _ _ _ _ w1152 _ _]
          seq-local: [_ _ _ _ _ _ _ _ _ _ w1139 _ _ _ _] -> [_ _ _ _ _ _ _ _ _ _ _ _ w1151 _ _]
          seq-local: [_ _ _ _ _ _ _ _ _ _ _ _ w1150 _ _] -> [_ _ _ _ _ _ _ _ _ _ _ _ _ _ w1163]
          seq-local: [_ _ _ _ _ _ _ _ _ _ _ _ w1149 _ _] -> [_ _ _ _ _ _ _ _ _ _ _ _ _ _ w1162]
          tunnel: w991 -> [w1093 _ _ _ _ _ _ _ _ _ _ _ _ _ _]
          tunnel: w992 -> [w1086 _ _ _ _ _ _ _ _ _ _ _ _ _ _]
          tunnel: w989 -> [w1085 _ w1099 _ w1106 _ w1122 _ w1133 _ w1143 _ w1153 _ w1166]
          tunnel: [_ _ _ _ _ _ _ _ _ _ _ _ _ _ w1161] -> w985
          tunnel: [_ _ _ _ _ _ _ _ _ _ _ _ _ _ w1160] -> w984
          frame #0 {
            w1090 = " PULSe"  # Function Command
            n404 = local read "输出信号波形"() -> (w1084:u16)
            n405 = Concatenate Strings(w1085, ":FUNC" ("string (\"\")")) -> (w1091:string)
            n406 = Pick Line(string ("")=w1091, multi-line string=w1090, line index=w1084) -> (output string=w1089:string)
            n407 = VISA Write(VISA resource name=w1093, write buffer=w1089, error in (no error)=w1086) -> (VISA resource name out=w1088:refnum<visa-resource-name>, error out=w1087:errorcluster)  [unwired: 1 out]
          }
          frame #1 {
            n408 = Wait (ms)(milliseconds to wait=u32 150) -> ()  [unwired: 1 out]
          }
          frame #2 {
            n409 = Number To Fractional String(use system decimal point (T)=TRUE ("使用系统小数点(T)"), number="低电平/V") -> (F-format string=w1097:string)  [unwired: 2 in]
            n410 = Concatenate Strings ("连接字符串")(w1099, ":VOLTage:LOW ", w1097) -> (w1096:string)
            n411 = VISA Write(VISA resource name=w1103, write buffer=w1096, error in (no error)=w1102) -> (VISA resource name out=w1101:refnum<visa-resource-name>, error out=w1100:errorcluster)  [unwired: 1 out]
          }
          frame #3 {
            n412 = Wait (ms)(milliseconds to wait=u32 150) -> ()  [unwired: 1 out]
          }
          frame #4 {
            # "1 频率"
            n413 = Concatenate Strings(w1106, ":FREQ ") -> (w1113:string)
            n414 = Format Into String ("格式化写入字符串")(initial string=w1113, "频率/Hz") -> (resulting string=w1114:string)  [unwired: 2 in, 1 out]
            n415 = VISA Write(VISA resource name=w1112, write buffer=w1114, error in (no error)=w1111) -> (VISA resource name out=w1110:refnum<visa-resource-name>, error out=w1107:errorcluster)  [unwired: 1 out]
          }
          frame #5 {
            n416 = Wait (ms)(milliseconds to wait=u32 150) -> ()  [unwired: 1 out]
          }
          frame #6 {
            n417 = Number To Fractional String(use system decimal point (T)=TRUE ("使用系统小数点(T)"), number="高电平/V") -> (F-format string=w1119:string)  [unwired: 2 in]
            n418 = Concatenate Strings(w1122, ":VOLTage:HIGH ", w1119) -> (w1121:string)
            n419 = VISA Write(VISA resource name=w1118, write buffer=w1121, error in (no error)=w1117) -> (VISA resource name out=w1125:refnum<visa-resource-name>, error out=w1124:errorcluster)  [unwired: 1 out]
          }
          frame #7 {
            n420 = Wait (ms)(milliseconds to wait=u32 150) -> ()  [unwired: 1 out]
          }
          frame #8 {
            n421 = local read "channel输出口"() -> (w1131:i32)
            n422 = Pick Line(multi-line string=":OUTP1:IMPedance \n:OUTP2:IMPedance " ("write buffer"), line index=w1131) -> (output string=w1130:string)  [unwired: 1 in]
            n423 = Concatenate Strings ("连接字符串")(w1133, w1130, "INFINITY") -> (w1134:string)
            n424 = VISA Write(VISA resource name=w1136, write buffer=w1134, error in (no error)=w1135) -> (VISA resource name out=w1129:refnum<visa-resource-name>, error out=w1128:errorcluster)  [unwired: 1 out]
          }
          frame #9 {
            n425 = Wait (ms)(milliseconds to wait=u32 150) -> ()  [unwired: 1 out]
          }
          frame #10 {
            n426 = Number To Fractional String(use system decimal point (T)=TRUE ("使用系统小数点(T)"), number="占空比/%") -> (F-format string=w1145:string)  [unwired: 2 in]
            n427 = Concatenate Strings(w1143, ":PULSe:DCYCle ", w1145) -> (w1140:string)
            n428 = VISA Write(VISA resource name=w1142, write buffer=w1140, error in (no error)=w1141) -> (VISA resource name out=w1138:refnum<visa-resource-name>, error out=w1139:errorcluster)  [unwired: 1 out]
          }
          frame #11 {
            n429 = Wait (ms)(milliseconds to wait=u32 150) -> ()  [unwired: 1 out]
          }
          frame #12 {
            n430 = Number To Fractional String(use system decimal point (T)=TRUE ("使用系统小数点(T)"), number="延时/s") -> (F-format string=w1156:string)  [unwired: 2 in]
            n431 = Concatenate Strings(w1153, ":PULSe:DELay ", w1156) -> (w1154:string)
            n432 = VISA Write(VISA resource name=w1152, write buffer=w1154, error in (no error)=w1151) -> (VISA resource name out=w1150:refnum<visa-resource-name>, error out=w1149:errorcluster)  [unwired: 1 out]
          }
          frame #13 {
            n433 = Wait (ms)(milliseconds to wait=u32 150) -> ()  [unwired: 1 out]
          }
          frame #14 {
            w1167 = ":LEADing\n:TRAiling "  # Channel
            w1172 = ":PULSe:TRANsition"  # VOLTage:Offset
            n434 = local read "上升下降沿"() -> (w1168:i32)
            n435 = Pick Line(multi-line string=w1167, line index=w1168) -> (output string=w1164:string)  [unwired: 1 in]
            n436 = Number To Fractional String(use system decimal point (T)=TRUE ("使用系统小数点(T)"), number="上升下降沿/s") -> (F-format string=w1165:string)  [unwired: 2 in]
            n437 = Concatenate Strings(w1166, w1172, w1164, w1165) -> (w1169:string)
            n438 = VISA Write(VISA resource name=w1163, write buffer=w1169, error in (no error)=w1162) -> (VISA resource name out=w1161:refnum<visa-resource-name>, error out=w1160:errorcluster)  [unwired: 1 out]
          }
        }
        n439 = stacked-sequence {
          seq-local: [w999 _ _ _ _ _ _ _ _ _ _ _ _ _ _] -> [_ _ w1014 _ _ _ _ _ _ _ _ _ _ _ _]
          seq-local: [w998 _ _ _ _ _ _ _ _ _ _ _ _ _ _] -> [_ _ w1013 _ _ _ _ _ _ _ w1052 _ _ _ _]
          seq-local: [_ _ w1012 _ _ _ _ _ _ _ _ _ _ _ _] -> [_ _ _ _ w1023 _ _ _ _ _ _ _ _ _ _]
          seq-local: [_ _ w1011 _ _ _ _ _ _ _ _ _ _ _ _] -> [_ _ _ _ w1022 _ _ _ _ _ _ _ _ _ _]
          seq-local: [_ _ _ _ w1021 _ _ _ _ _ _ _ _ _ _] -> [_ _ _ _ _ _ w1029 _ _ _ _ _ _ _ _]
          seq-local: [_ _ _ _ w1018 _ _ _ _ _ _ _ _ _ _] -> [_ _ _ _ _ _ w1028 _ _ _ _ _ _ _ _]
          seq-local: [_ _ _ _ _ _ w1036 _ _ _ _ _ _ _ _] -> [_ _ _ _ _ _ _ _ w1047 _ _ _ _ _ _]
          seq-local: [_ _ _ _ _ _ w1035 _ _ _ _ _ _ _ _] -> [_ _ _ _ _ _ _ _ w1046 _ _ _ _ _ _]
          seq-local: [_ _ _ _ _ _ _ _ w1041 _ _ _ _ _ _] -> [_ _ _ _ _ _ _ _ _ _ w1053 _ _ _ _]
          seq-local: [_ _ _ _ _ _ _ _ w1040 _ _ _ _ _ _] -> [_ _ _ _ _ _ _ _ _ _ _ _ _ _ _]
          seq-local: [_ _ _ _ _ _ _ _ _ _ w1049 _ _ _ _] -> [_ _ _ _ _ _ _ _ _ _ _ _ w1063 _ _]
          seq-local: [_ _ _ _ _ _ _ _ _ _ w1050 _ _ _ _] -> [_ _ _ _ _ _ _ _ _ _ _ _ w1062 _ _]
          seq-local: [_ _ _ _ _ _ _ _ _ _ _ _ w1061 _ _] -> [_ _ _ _ _ _ _ _ _ _ _ _ _ _ w1076]
          seq-local: [_ _ _ _ _ _ _ _ _ _ _ _ w1060 _ _] -> [_ _ _ _ _ _ _ _ _ _ _ _ _ _ w1075]
          tunnel: w985 -> [w1004 _ _ _ _ _ _ _ _ _ _ _ _ _ _]
          tunnel: w984 -> [w997 _ _ _ _ _ _ _ _ _ _ _ _ _ _]
          tunnel: w981 -> [w996 _ w1010 _ w1017 _ w1033 _ w1044 _ w1054 _ w1064 _ w1071]
          tunnel: [_ _ _ _ _ _ _ _ _ _ _ _ _ _ w1074] -> w983
          tunnel: [_ _ _ _ _ _ _ _ _ _ _ _ _ _ w1073] -> w982
          tunnel: w980 -> [_ _ _ _ _ _ _ _ w1038 _ _ _ _ _ _]
          frame #0 {
            w1001 = " PULSe"  # Function Command
            n440 = Concatenate Strings(w996, ":FUNC" ("string (\"\")")) -> (w1002:string)
            n441 = Pick Line(string ("")=w1002, multi-line string=w1001, line index="输出信号波形 2") -> (output string=w1000:string)
            n442 = VISA Write(VISA resource name=w1004, write buffer=w1000, error in (no error)=w997) -> (VISA resource name out=w999:refnum<visa-resource-name>, error out=w998:errorcluster)  [unwired: 1 out]
          }
          frame #1 {
            n443 = Wait (ms)(milliseconds to wait=u32 150) -> ()  [unwired: 1 out]
          }
          frame #2 {
            n444 = Number To Fractional String(use system decimal point (T)=TRUE ("使用系统小数点(T)"), number="低电平/V 2") -> (F-format string=w1008:string)  [unwired: 2 in]
            n445 = Concatenate Strings ("连接字符串")(w1010, ":VOLTage:LOW ", w1008) -> (w1007:string)
            n446 = VISA Write(VISA resource name=w1014, write buffer=w1007, error in (no error)=w1013) -> (VISA resource name out=w1012:refnum<visa-resource-name>, error out=w1011:errorcluster)  [unwired: 1 out]
          }
          frame #3 {
            n447 = Wait (ms)(milliseconds to wait=u32 150) -> ()  [unwired: 1 out]
          }
          frame #4 {
            # "1 频率"
            n448 = Concatenate Strings(w1017, ":FREQ ") -> (w1024:string)
            n449 = Format Into String ("格式化写入字符串")(initial string=w1024, "频率/Hz 2") -> (resulting string=w1025:string)  [unwired: 2 in, 1 out]
            n450 = VISA Write(VISA resource name=w1023, write buffer=w1025, error in (no error)=w1022) -> (VISA resource name out=w1021:refnum<visa-resource-name>, error out=w1018:errorcluster)  [unwired: 1 out]
          }
          frame #5 {
            n451 = Wait (ms)(milliseconds to wait=u32 150) -> ()  [unwired: 1 out]
          }
          frame #6 {
            n452 = Number To Fractional String(use system decimal point (T)=TRUE ("使用系统小数点(T)"), number="高电平/V 2") -> (F-format string=w1030:string)  [unwired: 2 in]
            n453 = Concatenate Strings(w1033, ":VOLTage:HIGH ", w1030) -> (w1032:string)
            n454 = VISA Write(VISA resource name=w1029, write buffer=w1032, error in (no error)=w1028) -> (VISA resource name out=w1036:refnum<visa-resource-name>, error out=w1035:errorcluster)  [unwired: 1 out]
          }
          frame #7 {
            n455 = Wait (ms)(milliseconds to wait=u32 150) -> ()  [unwired: 1 out]
          }
          frame #8 {
            n456 = Pick Line(multi-line string=":OUTP1:IMPedance \n:OUTP2:IMPedance " ("write buffer"), line index=w1038) -> (output string=w1042:string)  [unwired: 1 in]
            n457 = Concatenate Strings ("连接字符串")(w1044, w1042, "INFINITY") -> (w1045:string)
            n458 = VISA Write(VISA resource name=w1047, write buffer=w1045, error in (no error)=w1046) -> (VISA resource name out=w1041:refnum<visa-resource-name>, error out=w1040:errorcluster)  [unwired: 1 out]
          }
          frame #9 {
            n459 = Wait (ms)(milliseconds to wait=u32 150) -> ()  [unwired: 1 out]
          }
          frame #10 {
            n460 = Number To Fractional String(use system decimal point (T)=TRUE ("使用系统小数点(T)"), number="占空比/% 2") -> (F-format string=w1056:string)  [unwired: 2 in]
            n461 = Concatenate Strings(w1054, ":PULSe:DCYCle ", w1056) -> (w1051:string)
            n462 = VISA Write(VISA resource name=w1053, write buffer=w1051, error in (no error)=w1052) -> (VISA resource name out=w1049:refnum<visa-resource-name>, error out=w1050:errorcluster)  [unwired: 1 out]
          }
          frame #11 {
            n463 = Wait (ms)(milliseconds to wait=u32 150) -> ()  [unwired: 1 out]
          }
          frame #12 {
            n464 = Number To Fractional String(use system decimal point (T)=TRUE ("使用系统小数点(T)"), number="延时/s 2") -> (F-format string=w1067:string)  [unwired: 2 in]
            n465 = Concatenate Strings(w1064, ":PULSe:DELay ", w1067) -> (w1065:string)
            n466 = VISA Write(VISA resource name=w1063, write buffer=w1065, error in (no error)=w1062) -> (VISA resource name out=w1061:refnum<visa-resource-name>, error out=w1060:errorcluster)  [unwired: 1 out]
          }
          frame #13 {
            n467 = Wait (ms)(milliseconds to wait=u32 150) -> ()  [unwired: 1 out]
          }
          frame #14 {
            w1079 = ":LEADing\n:TRAiling "  # Channel
            w1083 = ":PULSe:TRANsition"  # VOLTage:Offset
            n468 = Pick Line(multi-line string=w1079, line index="上升下降沿 2") -> (output string=w1077:string)  [unwired: 1 in]
            n469 = Number To Fractional String(use system decimal point (T)=TRUE ("使用系统小数点(T)"), number="上升下降沿/s 2") -> (F-format string=w1078:string)  [unwired: 2 in]
            n470 = Concatenate Strings(w1071, w1083, w1077, w1078) -> (w1080:string)
            n471 = VISA Write(VISA resource name=w1076, write buffer=w1080, error in (no error)=w1075) -> (VISA resource name out=w1074:refnum<visa-resource-name>, error out=w1073:errorcluster)  [unwired: 1 out]
          }
        }
        n472 = VISA Close(VISA resource name=w983, error in (no error)=w982) -> (error out=→"configure error out":errorcluster)
      }
    }
    n473 = event shown="[1] \"照明光\": 值改变" {
      selector: _ -> [_ _]
      dyn-events: _ -> [_ _]
      timeout: 0 -> [_ _]
      tunnel: "照明光" -> [_ w61]
      event Timeout {
        n474 = event-data() -> ()  [unwired: 1 in, 3 out]
      }
      event "照明光": Value Change {
        n475 = event-data() -> ()  [unwired: 1 in, 6 out]
        n476 = local read "stop bits (10: 1 bit)"() -> (w74:u16)
        n477 = local read "parity (0:none)"() -> (w73:enum16{"None", "Odd", "Even", "Mark", "Space"})
        n478 = local read "照明光VISA"() -> (w70:refnum<visa-resource-name>)
        n479 = local read "baud rate"() -> (w71:u32)
        n480 = local read "data bits (8)"() -> (w72:u16)
        n481 = call-poly "VISA Configure Serial Port"("VISA resource name"=w70, "baud rate (9600)"=w71, "data bits (8)"=w72, "parity (0:none)"=w73, "stop bits (10: 1 bit)"=w74) -> ("VISA resource name out"=w67:refnum<visa-resource-name>, "error out"=w66:errorcluster)  [unwired: 9 in]
        n482 = call <vilib>:"Simple Error Handler.vi"("error in (no error)"=w66) -> ()  [unwired: 4 in, 5 out]
        n483 = VISA Open(access mode=0, error in (no error)=w66, VISA resource name=w67) -> (VISA resource name=w69:refnum<visa-resource-name>, error out=w68:errorcluster)  [unwired: 2 in]
        n484 = stacked-sequence {
          tunnel: w69 -> [w79]
          tunnel: w68 -> [w78]
          tunnel: [w77] -> w64
          tunnel: [w76] -> w65
          tunnel: w61 -> [w75]
          frame #0 {
            n485 = case shown="假" w75 {
              tunnel: w79 -> [w85 w95]
              tunnel: [w83 w94] -> w77
              tunnel: w78 -> [w84 w93]
              tunnel: [w82 w92] -> w76
              frame False {
                n486 = Concatenate Strings(" \u0001\u0001¢", "\r") -> (w86:string)
                n487 = VISA Write(VISA resource name=w85, write buffer=w86, error in (no error)=w84) -> (VISA resource name out=w83:refnum<visa-resource-name>, error out=w82:errorcluster)  [unwired: 1 out]
                n488 = Wait (ms)(milliseconds to wait=50) -> ()  [unwired: 1 out]
              }
              frame True {
                w88 = " \u0001\u0000¡"  # Channel
                n489 = Wait (ms)(milliseconds to wait=50) -> ()  [unwired: 1 out]
                n490 = Concatenate Strings(w88, "\r") -> (w89:string)
                n491 = VISA Write(VISA resource name=w95, write buffer=w89, error in (no error)=w93) -> (VISA resource name out=w94:refnum<visa-resource-name>, error out=w92:errorcluster)  [unwired: 1 out]
              }
            }
          }
        }
        n492 = VISA Close(VISA resource name=w64, error in (no error)=w65) -> (error out=w63:errorcluster)
        n493 = call <vilib>:"Simple Error Handler.vi"("error in (no error)"=w63) -> ()  [unwired: 4 in, 5 out]
      }
    }
  }
  n494 = flat-sequence {
    frame #0 {
      "Backlight" <- i32[][] [] ("Backlight")
    }
    frame #1 {
      w1174 = FALSE
      # "删除背景光控件\n初始值设定"
      n495 = local write "cut backlight"(w1174) -> ()
      "backlight" <- w1174
    }
  }
  n496 = stacked-sequence {
    seq-local: [_ _ _ w1195 _ _ _ _] -> [_ _ _ _ w1213 w1233 w1236 w1438]
    seq-local: [_ _ _ w1194 _ _ _ _] -> [_ _ _ _ w1214 w1234 w1235 w1439]
    frame #0 {
      # "initialize all variables"
      n497 = property on="initialize" class="Bool"("Désactivé"=u8 0) -> ()  [unwired: 2 in, 2 out]
      n498 = property on="Acquire" class="Bool"("Visible"=FALSE) -> ()  [unwired: 2 in, 2 out]
      n499 = property on="Setup" class="Bool"("Visible"=FALSE) -> ()  [unwired: 2 in, 2 out]
      n500 = local write "indicator"("" ("indicator")) -> ()
      n501 = local write "initialized ?"(FALSE ("initialized ?")) -> ()
      n502 = local write "Continuous"(FALSE ("Continuous")) -> ()
      n503 = local write "Close"(FALSE ("Close")) -> ()
      n504 = property on="Device Name" class="Ring (严格)"("Désactivé"=u8 0) -> ()  [unwired: 2 in, 2 out]
      n505 = property on="Continuous" class="Bool (严格)"("Visible"=FALSE) -> ()  [unwired: 2 in, 2 out]
      n506 = local write "Commande tab"(T1."Settings" ("Commande tab")) -> ()
    }
    frame #1 {
      # "Read Uniq ID"
      n507 = stacked-sequence {
        frame #0 {
          n508 = call "read detector uniq-id.vi"() -> ("nbr of components"=w1187:i32, "UniqueID"=w1186:string[], "Name"=w1185:string[])  [unwired: 4 out]
          n509 = for {
            N: w1187 -> [_]
            tunnel: w1186 -> [w1189]
            tunnel: w1185 -> [w1188]
            n510 = property on="Device Name" class="Ring (严格)"("Chaînes []"=w1188) -> ()  [unwired: 2 in, 2 out]
            n511 = property on="Uniques ID" class="Ring (严格)"("Chaînes []"=w1189) -> ()  [unwired: 2 in, 2 out]
          }
        }
      }
    }
    frame #2 {
      n512 = while {
        stop <- "initialize" stop-if-true
        n513 = local read "Device Name"() -> (w1192:u16)
        n514 = local write "Uniques ID"(w1192) -> ()
        n515 = local read "Close"() -> (w1190:bool)
        n516 = Stop(stop? (T)=w1190) -> ()
        n517 = Wait Until Next ms Multiple(millisecond multiple=u32 100 ("n millisecondes")) -> ()  [unwired: 1 out]
      }
    }
    frame #3 {
      n518 = stacked-sequence {
        tunnel: [_ w1202 _ _] -> w1195
        tunnel: [_ w1201 _ _] -> w1194
        frame #0 {
          n519 = local write "indicator"("Initializing ..." ("indicator")) -> ()
        }
        frame #1 {
          n520 = local read "Uniques ID"() -> (w1199:u16)
          n521 = property on="Uniques ID" class="Ring (严格)"() -> ("Chaînes []"=w1200:string[])  [unwired: 2 in, 2 out]
          n522 = Index Array(array=w1200, index=w1199) -> (element=w1198:string)
          n523 = call "Initialize CCD.vi"("Unique id:"=w1198) -> ("activeYPixels"=→"Y Pixels:":i32, "JYCCDLib.IJYCCDReqd"=w1201:refnum<k7>, "activeXPixels"=→"X Pixels:":i32, "sortie d'erreur"=w1202:errorcluster, "FirmwareVersion"=→"Firmware\nVersion":string)  [unwired: 3 out]
        }
        frame #2 {
          n524 = property on="initialize" class="Bool"("Désactivé"=u8 2) -> ()  [unwired: 2 in, 2 out]
          n525 = property on="Device Name" class="Ring (严格)"("Désactivé"=u8 2) -> ()  [unwired: 2 in, 2 out]
          n526 = local write "Continuous"(FALSE ("Continuous")) -> ()
          n527 = property on="Setup" class="Bool"("Visible"=TRUE) -> ()  [unwired: 2 in, 2 out]
        }
        frame #3 {
          n528 = local write "initialized ?"(TRUE ("initialized ?")) -> ()
          n529 = local write "indicator"("Initialized !" ("indicator")) -> ()
        }
      }
    }
    frame #4 {
      # "Actually not working"
      # "Read ADC and GAIN"
      n530 = case shown="真" "Constante de condition\n(Voir l'aide contextuelle)" {
        tunnel: w1214 -> [_ w1224]
        tunnel: w1213 -> [_ w1223]
        frame False {
        }
        frame True {
          # "Read Input supported trigger"
          n531 = call "Trigger - Get Supported Input.vi"("JYCCDLib.IJYCCDReqd"=w1224, "Error Input"=w1223) -> ("trigAddress"=w1218:i32, "eventPtr"=w1219:i32, "trigEventString"=w1222:string, "trigSigType"=w1221:i32, "trigSigTypeString"=w1220:string)  [unwired: 4 out]
          n532 = local write "trigSigTypeString"(w1220) -> ()
          n533 = local write "trigAddress"(w1218) -> ()
          n534 = local write "Trigger Type :"(w1219) -> ()
          n535 = local write "trigEventString"(w1222) -> ()
          n536 = local write "Signal type :"(w1221) -> ()
        }
      }
      n537 = call "Init ADC & Gain.vi"("JYCCDLib.IJYCCDReqd"=w1214, "input error"=w1213) -> ("ADC Number"=w1212:i32[], "ADC description"=w1217:string[], "Gain Number"=w1215:i32[], "Gain description"=w1216:string[])
      n538 = local write "Gain Number"(w1215) -> ()
      n539 = local write "ADC Number"(w1212) -> ()
      n540 = stacked-sequence {
        tunnel: w1217 -> [w1225 _]
        tunnel: w1216 -> [_ w1226]
        frame #0 {
          n541 = property on="ADC" class="Ring (严格)"("Chaînes []"=w1225) -> ()  [unwired: 2 in, 2 out]
        }
        frame #1 {
          n542 = property on="GAIN" class="Ring (严格)"("Chaînes []"=w1226) -> ()  [unwired: 2 in, 2 out]
        }
      }
    }
    frame #5 {
      # "IS multi Accumulation Supported ?"
      n543 = call "MultiAccu - Is Supported.vi"("Error In"=w1233, "JYCCDLib.IJYCCDReqd"=w1234) -> ("IsOperatingModeSupported"=w1227:bool)  [unwired: 3 out]
      n544 = Select(t=0, s=w1227, f=2) -> (s? t:f=w1230:i32)
      n545 = Select(t=FALSE, s=w1227, f=w1227) -> (s? t:f=w1229:bool)
      n546 = local write "Multi Accumulation mode:"(w1229) -> ()
      n547 = property on="Multi Accumulation mode:" class="Bool (严格)"("Désactivé"=w1230) -> ()  [unwired: 2 in, 2 out]
      n548 = property on="Multi Accumulation mode:" class="Bool (严格)"("Désactivé"=w1230) -> ()  [unwired: 2 in, 2 out]
    }
    frame #6 {
      n549 = while {
        tunnel: w1235 -> [w1243]
        tunnel: w1236 -> [w1242]
        stop <- "Close" stop-if-true
        n550 = local read "Continuous"() -> (w1244:bool)
        n551 = case shown="假" "Reformat" {
          frame False {
          }
          frame True {
            n552 = local read "Y Pixels:"() -> (w1416:i32)
            n553 = local read "X Pixels:"() -> (w1418:i32)
            n554 = call "Spectral Reformat CCD area.vi"("Y Pixels:"=w1416, "X Pixels:"=w1418, "numAreas"="Number of Areas :") -> ("areas :"=→"areas :":i32[][])  [unwired: 3 out]
          }
        }
        n555 = local read "Accumulations:"() -> (w1239:u16)
        n556 = Or(x="Acquire", y=w1244) -> (x .or. y?=w1241:bool)
        n557 = case shown="真" w1241 {
          tunnel: w1243 -> [_ w1256]
          tunnel: w1242 -> [_ w1255]
          tunnel: "Enable InputTriggers :" -> [_ w1254]
          tunnel: "Multi Accumulation mode:" -> [_ w1253]
          tunnel: w1239 -> [_ w1252]
          tunnel: "MultiAcqShutterMode" -> [_ w1251]
          frame False {
          }
          frame True {
            n558 = stacked-sequence {
              seq-local: [_ _ w1269 _ _] -> [_ _ _ w1342 _]
              seq-local: [_ _ _ w1315 _] -> [_ _ _ _ w1382]
              tunnel: w1256 -> [_ w1258 w1273 w1341 _]
              tunnel: w1255 -> [_ w1259 w1272 w1340 _]
              tunnel: w1254 -> [_ w1260 _ _ _]
              tunnel: w1253 -> [_ _ w1271 _ _]
              tunnel: w1252 -> [_ _ w1270 _ _]
              tunnel: w1251 -> [_ _ w1268 _ _]
              frame #0 {
                n559 = local write "CCD Busy"(TRUE ("CCD Busy")) -> ()
              }
              frame #1 {
                n560 = case shown="真" w1260 {
                  tunnel: w1259 -> [w1261 w1267]
                  tunnel: w1258 -> [w1262 w1266]
                  frame False {
                    n561 = call "Trigger - Disable.vi"("Error In"=w1261, "JYCCDLib.IJYCCDReqd"=w1262) -> ()  [unwired: 6 out]
                  }
                  frame True {
                    n562 = local read "Trigger Type :"() -> (w1263:u16)
                    n563 = local read "Signal type :"() -> (w1264:enum16{"TTL Rising Edge", "TTL Falling Edge"})
                    n564 = local read "trigAddress"() -> (w1265:i32)
                    n565 = call "Trigger - Enable.vi"("Error In"=w1267, "sigType"=w1264, "event"=w1263, "trigAddress"=w1265, "JYCCDLib.IJYCCDReqd"=w1266) -> ()  [unwired: 3 out]
                  }
                }
              }
              frame #2 {
                n566 = case shown="真" w1271 {
                  selector: w1271 -> [_ w1302]
                  tunnel: w1273 -> [w1299 w1305]
                  tunnel: w1272 -> [w1298 w1304]
                  tunnel: w1270 -> [_ w1303]
                  tunnel: [u16 1 ("Accumulations:") w1303] -> w1269
                  tunnel: w1268 -> [_ w1301]
                  frame False {
                    n567 = call "MultiAccu - Disable.vi"("Error In"=w1298, "JYCCDLib.IJYCCDReqd"=w1299) -> ()  [unwired: 4 out]
                  }
                  frame True {
                    n568 = call "MultiAccu - Configure.vi"("JYCCDLib.IJYCCDReqd"=w1305, "Cleans Before"="Number of Cleans", "Accumulations:"=w1303, "MultiAcqHardwareMode"=w1302, "MultiAcqShutterMode"=w1301, "Error In"=w1304) -> ()  [unwired: 1 in, 9 out]
                  }
                }
                n569 = flat-sequence {
                  frame #0 {
                    n570 = Current VI's Path() -> (path=w1279:path)
                    n571 = Get Date/Time In Seconds() -> (seconds since 1Jan1904=w1281:timestamp)
                    n572 = Strip Path(path=w1279) -> (stripped path=w1280:path)  [unwired: 1 out]
                    n573 = Path To String(path=w1280) -> (string=w1282:string)
                    n574 = Format Date/Time String(time format string (%c)="%m.%d" ("时间格式字符串(%c)"), seconds (now)=w1281) -> (date/time string=w1288:string)  [unwired: 1 in]
                    n575 = Concatenate Strings(w1282, "\\Save\\" ("字符串"), w1288) -> (w1283:string)
                    n576 = String To Path(string=w1283) -> (path=w1284:path)
                    n577 = call <vilib>:"Check if File or Folder Exists.vi"("path"=w1284) -> ("file or folder exists?"=w1285:bool, "dup path"=w1287:path)  [unwired: 8 in, 1 out]
                    n578 = case shown="真" w1285 {
                      tunnel: [w1295 w1296] -> w1286
                      tunnel: w1287 -> [w1294 w1296]
                      tunnel: w1288 -> [w1293 _]
                      frame False {
                        n579 = Create Folder(prompt (Create Folder)=w1293, path (use dialog)=w1294) -> (created path=w1295:path)  [unwired: 1 in, 2 out]
                      }
                      frame True {
                      }
                    }
                    n580 = Format Date/Time String(time format string (%c)="%y%m%d%H%M%S " ("时间格式字符串(%c)"), seconds (now)=w1281) -> (date/time string=w1291:string)  [unwired: 1 in]
                    n581 = Path To String(path=w1286) -> (string=w1289:string)
                    n582 = Concatenate Strings(w1289, "\\" ("字符串")) -> (w1290:string)
                    n583 = Concatenate Strings(w1290, w1291) -> (w1278:string)
                    n584 = String To Path(string=w1278) -> (path=→"最终存储路径 2":path)
                  }
                }
              }
              frame #3 {
                n585 = local read "cut backlight"() -> (w1329:bool)
                n586 = local read "backlight"() -> (w1328:bool)
                n587 = call "MultiAccu - Acquire spectral.vi"("error in"=w1340, "Accumulations:"=w1342, "ShutterOpen"="ShutterOpen", "JYCCDLib.IJYCCDReqd"=w1341) -> ("Acq Time(ms)"=→"Acq Time(ms)":u32, "Array Out"=w1339:i32[][][])  [unwired: 1 out]
                n588 = And(x=w1329, y=w1328) -> (x .and. y?=w1330:bool)
                n589 = call "Array reset dimension.vi"("Area Number"="Area Number to Display", "Array In"=w1339) -> ("Array Out"=w1331:i32[][])
                n590 = case shown="真" w1330 {
                  tunnel: [w1378 w1379] -> w1332
                  tunnel: w1331 -> [w1378 w1380]
                  frame False {
                  }
                  frame True {
                    n591 = local read "Backlight"() -> (w1381:i32[][])
                    n592 = Subtract(x=w1380, y=w1381) -> (x-y=w1379:i32[][])
                  }
                }
                n593 = local read "波长范围"() -> (w1307:dbl[])
                n594 = local write "Data"(w1331) -> ()
                n595 = Index Array(array=w1332, index (row)=0 ("禁用的索引 (列)")) -> (element=w1333:i32[])  [unwired: 1 in]
                n596 = Reverse 1D Array(array=w1333) -> (reversed array=w1316:i32[])
                n597 = call "转换至动态数据2"("Array"=w1307) -> ("Dynamic Data Type"=w1335:dynamicdata)  [unwired: 3 in]
                n598 = call "转换至动态数据"("Array"=w1316) -> ("Dynamic Data Type"=w1336:dynamicdata)  [unwired: 3 in]
                n599 = call <vilib>:"Median Filter.vi"("left rank"=6, "X"=w1316) -> ("Filtered X"=w1321:dbl[])  [unwired: 8 in, 1 out]
                n600 = call "Build XY Graph"("Y Input"=w1336, "X Input"=w1335) -> ("XY Graph"=w1334:cluster{"Y":dbl[], "Y":dbl[]}[])  [unwired: 8 in, 1 out]
                n601 = Subtract(x="拟合终点", y="拟合起点") -> (x-y=w1310:i32)
                n602 = local write "Spectrum"(w1334) -> ()
                n603 = local read "滤波阈值"() -> (w1325:dbl)
                n604 = Array Subset(array=w1307, index="拟合起点", length=w1310) -> (w1313:dbl[])
                n605 = local read "拟合参数"() -> (w1306:dbl[])
                n606 = In Range and Coerce(upper limit=w1325, x=w1321, lower limit=-100.0) -> (In Range?=w1324:bool[])  [unwired: 1 out]
                n607 = Not(x=w1324) -> (.not. x?=w1318:bool[])
                n608 = local read "滤波阈值"() -> (w1320:dbl)
                n609 = local write "范围内？"(w1324) -> ()
                n610 = local read "X Pixels:"() -> (w1322:i32)
                n611 = Or Array Elements(Boolean array=w1318) -> (logical OR=w1323:bool)
                n612 = case shown="真" w1323 {
                  tunnel: w1322 -> [_ w1365]
                  tunnel: w1321 -> [w1361 w1364]
                  tunnel: [w1361 w1363] -> w1309
                  tunnel: w1320 -> [_ w1362]
                  frame False {
                  }
                  frame True {
                    n613 = for {
                      N: w1365 -> [_]
                      tunnel: w1364 -> [w1369] mode=indexing
                      tunnel: [w1368] -> w1363 mode=indexing
                      shift-right: [w1368] -> _
                      shift-left: _ -> [w1367]
                      tunnel: w1362 -> [w1366]
                      n614 = Greater?(x=w1369, y=w1366) -> (0:w1371:bool)
                      n615 = Less?(x=w1369, y=-100.0) -> (x < y?=w1372:bool)
                      n616 = Or(x=w1371, y=w1372) -> (x .or. y?=w1370:bool)
                      n617 = case shown="真" w1370 {
                        tunnel: w1369 -> [w1374 _]
                        tunnel: [w1374 w1376] -> w1368
                        tunnel: w1367 -> [_ w1377]
                        frame False {
                        }
                        frame True {
                          n618 = call <vilib>:"Median Filter PtByPt.vi"("rank"=5, "x"=w1377) -> ("Filtered x"=w1376:dbl)  [unwired: 2 in, 1 out]
                        }
                      }
                    }
                  }
                }
                n619 = Array Subset(array=w1309, index="拟合起点", length=w1310) -> (w1312:dbl[])
                n620 = Bundle("波长范围"=w1307, "Filtered X"=w1309) -> (w1308:cluster{"波长范围 ":dbl[], "Filtered X":dbl[]})  [unwired: 1 in]
                n621 = case shown="真" "是否拟合" {
                  tunnel: w1312 -> [w1345 w1351]
                  tunnel: w1313 -> [_ w1350]
                  tunnel: [w1345 w1349] -> w1327
                  tunnel: w1308 -> [_ w1347]
                  frame False {
                  }
                  frame True {
                    n622 = call "转换至动态数据3"("Array"=w1351) -> ("Dynamic Data Type"=w1356:dynamicdata)  [unwired: 3 in]
                    n623 = call "转换至动态数据4"("Array"=w1350) -> ("Dynamic Data Type"=w1357:dynamicdata)  [unwired: 3 in]
                    n624 = call "曲线拟合"("Locations"=w1357, "Signals"=w1356) -> ("best fit"=w1354:dynamicdata, "non-linear coefficients"=w1355:dynamicdata)  [unwired: 5 in, 3 out]
                    n625 = call "从动态数据转换"("Dynamic Data Type"=w1355) -> ("Array"=w1358:dbl[])  [unwired: 3 in]
                    n626 = call "从动态数据转换2"("Dynamic Data Type"=w1354) -> ("Array"=w1349:dbl[])  [unwired: 3 in]
                    n627 = Index Array(array=w1358, index #1=0 ("索引"), index #2=1 ("索引")) -> (element #1=w1360:dbl, element #2=w1359:dbl)
                    n628 = local write "拟合参数"(w1358) -> ()
                    n629 = local write "xc"(w1360) -> ()
                    n630 = Bundle(w1350, "Array"=w1349) -> (w1348:cluster{dbl[], "Array":dbl[]})  [unwired: 1 in]
                    n631 = local write "w"(w1359) -> ()
                    n632 = Build Array(w1347, w1348) -> (→"best fit":cluster{"波长范围 ":dbl[], "Array":dbl[]}[])
                  }
                }
                n633 = Build Array(w1313, w1316, w1327, w1306) -> (w1315:dbl[][])
              }
              frame #4 {
                n634 = case shown="真" "是否保存" {
                  tunnel: w1382 -> [_ w1386]
                  frame False {
                  }
                  frame True {
                    n635 = Get Date/Time In Seconds() -> (seconds since 1Jan1904=w1400:timestamp)
                    n636 = Get Date/Time String(date format (0)=enum16{"short", "long", "abbreviated"}."abbreviated" ("日期格式(0)"), seconds (now)=w1400, want seconds? (F)=TRUE ("需要秒？(F)")) -> (date string=w1398:string, time string=w1399:string)
                    n637 = Search and Replace String(replace all?=TRUE ("替换全部？(F)"), input string=w1399, search string=":" ("搜索字符串"), replace string="-" ("替换字符串(\"\")")) -> (result string=w1397:string)  [unwired: 4 in, 3 out]
                    n638 = local read "最终存储路径 2"() -> (w1401:path)
                    n639 = Path To String(path=w1401) -> (string=w1404:string)
                    n640 = Concatenate Strings(w1404, w1398, w1397, "光谱" ("字符串"), ".xls" ("字符串")) -> (w1403:string)
                    n641 = String To Path(string=w1403) -> (path=w1402:path)
                    n642 = call-poly <vilib>:"Write Delimited Spreadsheet.vi"("file path (dialog if empty)"=w1402, "format (%.3f)"="%.16f", "2D data"=w1386, "append to file? (new file:F)"=TRUE ("append to file? (F)"), "transpose? (no:F)"=TRUE ("transpose? (F)")) -> ()  [unwired: 9 in, 2 out]
                  }
                }
                n643 = case shown="真" "Save Backlight" {
                  frame False {
                  }
                  frame True {
                    w1405 = TRUE ("删除背景光")
                    n644 = local read "Data"() -> (w1407:i32[][])
                    n645 = local write "Backlight"(w1407) -> ()
                    n646 = local write "cut backlight"(w1405) -> ()
                    n647 = local write "backlight"(w1405) -> ()
                    n648 = local write "Save Backlight"(FALSE ("Save Backlight")) -> ()
                  }
                }
                n649 = local write "CCD Busy"(FALSE ("CCD Busy")) -> ()
              }
            }
          }
        }
        n650 = case shown="真" "Setup" {
          tunnel: w1242 -> [_ w1421]
          tunnel: w1243 -> [_ w1420]
          frame False {
          }
          frame True {
            n651 = stacked-sequence {
              tunnel: w1421 -> [_ w1435 _]
              tunnel: w1420 -> [_ w1423 _]
              frame #0 {
                n652 = local write "indicator"("Setting up the detector" ("indicator")) -> ()
              }
              frame #1 {
                w1433 = 1 items=["JYMCD_ACQ_FORMAT_IMAGE", "JYMCD_ACQ_FORMAT_SCAN"] ("Acquisition type")
                n653 = local read "Gain Number"() -> (w1428:i32[])
                n654 = local read "GAIN"() -> (w1424:u16)
                n655 = local read "ADC Number"() -> (w1429:i32[])
                n656 = local read "ADC"() -> (w1425:u16)
                n657 = Index Array(array=w1428, index=w1424) -> (element=w1426:i32)
                n658 = Index Array(array=w1429, index=w1425) -> (element=w1427:i32)
                n659 = local read "Number of Areas :"() -> (w1431:u16)
                n660 = local read "areas :"() -> (w1432:i32[][])
                n661 = call "Setup CCD.vi"("numAreas"=w1431, "areas :"=w1432, "JYCCDLib.IJYCCDReqd"=w1423, "entrée d'erreur (pas d'erreur)"=w1435, "Acquisition type"=w1433, "Gain"=w1426, "Select ADC"=w1427, "Integration time(ms)"="Integration time (ms) :") -> ("DataSize"=→"DataSize":i32)  [unwired: 1 out]
                "JYCCDLib.IJYCCDReqd" <- w1423
              }
              frame #2 {
                w1436 = TRUE ("Visible")
                n662 = property on="Continuous" class="Bool (严格)"("Visible"=w1436) -> ()  [unwired: 2 in, 2 out]
                n663 = property on="Acquire" class="Bool"("Visible"=w1436) -> ()  [unwired: 2 in, 2 out]
                n664 = local write "indicator"("Ready !" ("indicator")) -> ()
              }
            }
          }
        }
        n665 = case shown="假" "Temperature" {
          tunnel: w1243 -> [_ w1410]
          tunnel: w1242 -> [_ w1409]
          frame False {
            n666 = property on="temp graph" class="WFChart (严格)"("Visible"=FALSE) -> ()  [unwired: 2 in, 2 out]
          }
          frame True {
            n667 = stacked-sequence {
              tunnel: w1410 -> [_ w1415]
              tunnel: w1409 -> [_ w1414]
              frame #0 {
                n668 = property on="temp graph" class="WFChart (严格)"("Visible"=TRUE) -> ()  [unwired: 2 in, 2 out]
              }
              frame #1 {
                w1413 = u16 0 items=["° Celsius", "Kelvin", "° Farenheit"] ("units")
                n669 = call "read temperature.vi"("entrée d'erreur (pas d'erreur)"=w1414, "units"=w1413, "JYCCDLib.IJYCCDReqd"=w1415) -> ("Current Temperature"=w1412:dbl)
                n670 = local write "temp graph"(w1412) -> ()
              }
            }
          }
        }
        n671 = Wait Until Next ms Multiple(millisecond multiple=u32 50 ("n millisecondes")) -> ()  [unwired: 1 out]
      }
    }
    frame #7 {
      n672 = Close Reference(reference=w1439, error in (no error)=w1438) -> ()  [unwired: 1 out]
    }
  }
  n673 = stacked-sequence {
    seq-local: [_ _ w1449 _ _] -> [_ _ _ w1459 w1464]
    seq-local: [_ _ w1448 _ _] -> [_ _ _ w1458 _]
    seq-local: [_ _ _ w1457 _] -> [_ _ _ _ _]
    frame #0 {
      n674 = call "Get Monos From Config Browser.vi"() -> ("UniqueIDs"=w1444:string[], "Mono ID"=w1445:string[])  [unwired: 3 in, 1 out]
      n675 = Build Cluster Array(w1445, w1444) -> (w1442:cluster{"String":string, "String":string}[])
      n676 = property on="Mono ID" class="CmbBox"("Strings And Values []"=w1442) -> ()  [unwired: 2 in, 2 out]
      n677 = Index Array(array=w1442, index=0) -> (element=w1443:cluster{"String":string, "String":string})
      n678 = Unbundle(w1443) -> ("String"=w1440:string)  [unwired: 1 out]
      "Current UniqueID" <- w1440
      n679 = local write "Mono ID"(w1440) -> ()
    }
    frame #1 {
      n680 = while {
        stop <- "Connect" stop-if-true
        n681 = local read "Mono ID"() -> (w1446:string)
        n682 = local write "Current UniqueID"(w1446) -> ()
      }
    }
    frame #2 {
      n683 = local read "Mono ID"() -> (w1451:string)
      n684 = call "JYInitMono.vi"("Unique ID"=w1451, "Force Init"="Force\nInitialization") -> ("Refnum out"=w1449:refnum<k7>, "Initialized"=→"Initialized JY":bool, "error out"=w1448:errorcluster)  [unwired: 9 in, 2 out]
    }
    frame #3 {
      n685 = call "Show Current Grating.vi"("Refnum in"=w1459, "error in (no error)"=w1458) -> ("Gratings"=w1460:dbl[], "Grating Index"=w1454:i32, "Current Grating"=w1456:dbl, "Current Description"=w1453:string, "error out"=w1457:errorcluster)  [unwired: 5 in, 4 out]
      "Gratings" <- w1460
      n686 = local write "Current Grating"(w1456) -> ()
      n687 = local write "Current Description"(w1453) -> ()
      n688 = Number To Decimal String(number=w1460) -> (decimal integer string=w1462:string[])  [unwired: 1 in]
      n689 = Number To Decimal String(number=w1454) -> (decimal integer string=w1455:string)  [unwired: 1 in]
      n690 = property on="Target Grating" class="CmbBox"("Value"=w1455) -> ()  [unwired: 2 in, 2 out]
      n691 = Build Cluster Array(w1462, string[] ["1", "2", "3"]) -> (w1463:cluster{"Numeric":string, string}[])
      n692 = property on="Target Grating" class="CmbBox"("Strings And Values []"=w1463) -> ()  [unwired: 2 in, 2 out]
    }
    frame #4 {
      n693 = while {
        tunnel: w1464 -> [w1466]
        stop <- w1465 stop-if-true
        n694 = stacked-sequence {
          seq-local: [w1470 _ _ _ _] -> [_ w1477 w1488 _ w1496]
          seq-local: [w1469 _ _ _ _] -> [_ w1476 w1487 _ _]
          seq-local: [_ w1475 _ _ _] -> [_ _ _ _ _]
          seq-local: [_ w1474 _ _ _] -> [_ _ _ _ _]
          seq-local: [_ _ w1480 _ _] -> [_ _ _ _ _]
          seq-local: [_ _ w1479 _ _] -> [_ _ _ w1490 _]
          tunnel: w1466 -> [w1468 _ _ w1491 _]
          frame #0 {
            n695 = call "Show Current Grating.vi"("Refnum in"=w1468) -> ("Grating Index"=→"Grating Index":i32, "Current Grating"=→"Current Grating":dbl, "Current Description"=→"Current Description":string, "error out"=w1469:errorcluster, "JYMONOLib.IJYMonoReqd"=w1470:refnum<k7>)  [unwired: 6 in, 4 out]
          }
          frame #1 {
            n696 = call "JYGetCurrentWL.vi"("error in (no error)"=w1476, "JYMONOLib.IJYMonoReqd"=w1477) -> ("error out"=w1474:errorcluster, "Units"=→"Units":string, "Current WL"=→"Current WL":dbl, "JYMONOLib.IJYMonoReqd 2"=w1475:refnum<k7>)  [unwired: 6 in]
          }
          frame #2 {
            w1485 = u16 1 items=["Entrance", "Exit"] ("Mirror Number")
            w1486 = u16 0 items=["Entrance", "Exit"] ("Mirror Number")
            n697 = call "JYGetMirrorPos.vi"("error in (no error)"=w1487, "Mirror"=w1486, "Refnum In"=w1488) -> ("error out"=w1483:errorcluster, "Current Mirror Position"=→"Entrance Mirror\nPosition":i32, "Refnum Out"=w1484:refnum<k7>)  [unwired: 1 in]
            n698 = call "JYGetMirrorPos.vi"("error in (no error)"=w1483, "Mirror"=w1485, "Refnum In"=w1484) -> ("error out"=w1479:errorcluster, "Current Mirror Position"=→"Exit Mirror\nPosition":i32, "Refnum Out"=w1480:refnum<k7>)  [unwired: 1 in]
          }
          frame #3 {
            w1493 = u16 0 items=["Front Entrance", "Side Entrance", "Front Exit", "Side Exit", "First Intermediate", "Second Intermediate"] ("Slit")
            n699 = call "JYGetSlits.vi"("MonoRefNum IN"=w1491, "Slit"=w1493, "error in (no error)"=w1490) -> ("Units"=→"Units 2":string, "Slit Width"=→"Front Entrance":dbl, "error out"=→"error out":errorcluster)  [unwired: 13 in, 1 out]
          }
          frame #4 {
            n700 = case shown="假" "Move To\nTarget Positions" {
              tunnel: w1496 -> [_ w1497]
              frame False {
              }
              frame True {
                n701 = stacked-sequence {
                  seq-local: [w1499 _ _ _] -> [_ w1505 _ _]
                  seq-local: [_ w1503 _ _] -> [_ _ w1520 _]
                  seq-local: [_ _ w1507 _] -> [_ _ _ w1526]
                  seq-local: [_ _ _ w1523] -> [_ _ _ _]
                  tunnel: w1497 -> [w1501 w1504 w1518 w1527]
                  frame #0 {
                    n702 = property on="Target Grating" class="CmbBox"() -> ("Value"=w1498:string)  [unwired: 2 in, 2 out]
                    n703 = local read "error out"() -> (w1500:errorcluster)
                    n704 = Decimal String To Number(string=w1498) -> (number=w1502:i32)  [unwired: 2 in, 1 out]
                    n705 = call "JYTurret.vi"("error in (no error)"=w1500, "Grating Index"=w1502, "JYMONOLib.IJYMonoReqd"=w1501) -> ("error out"=w1499:errorcluster)  [unwired: 2 out]
                  }
                  frame #1 {
                    # "Move Grating to Target Position"
                    n706 = call "JYMoveToWavelength.vi"("error in (no error)"=w1505, "Target WL"="Target WL", "RefNum In"=w1504) -> ("error out"=w1503:errorcluster)  [unwired: 1 in, 2 out]
                  }
                  frame #2 {
                    w1513 = u16 1 items=["Entrance", "Exit"] ("Mirror Number")
                    w1512 = u16 0 items=["Entrance", "Exit"] ("Mirror Number")
                    w1519 = u16 1 items=["Entrance", "Exit", "Front", "Side"] ("Mirror Number")
                    w1522 = u16 0 items=["Entrance", "Exit", "Front", "Side"] ("Mirror Number")
                    # "Move Mirrors"
                    n707 = call "JYMirrorMove.vi"("error in (no error)"=w1520, "Mirror Position"="Entrance Mirror", "Mirror Number"=w1522, "RefNum In"=w1518) -> ("error out"=w1517:errorcluster)  [unwired: 6 in, 1 out]
                    n708 = call "JYMirrorMove.vi"("error in (no error)"=w1517, "Mirror Position"="Exit Mirror", "Mirror Number"=w1519, "RefNum In"=w1518) -> ("error out"=w1510:errorcluster, "MonoRefNum Out"=w1511:refnum<k7>)  [unwired: 6 in]
                    n709 = call "JYGetMirrorPos.vi"("error in (no error)"=w1510, "Mirror"=w1512, "Refnum In"=w1511) -> ("error out"=w1515:errorcluster, "Current Mirror Position"=w1509:i32, "Refnum Out"=w1514:refnum<k7>)  [unwired: 1 in]
                    n710 = local write "Entrance Mirror\nPosition"(w1509) -> ()
                    n711 = call "JYGetMirrorPos.vi"("error in (no error)"=w1515, "Mirror"=w1513, "Refnum In"=w1514) -> ("error out"=w1507:errorcluster, "Current Mirror Position"=w1508:i32)  [unwired: 1 in, 1 out]
                    n712 = local write "Exit Mirror\nPosition"(w1508) -> ()
                  }
                  frame #3 {
                    w1525 = u16 0 items=["Front Entrance", "Side Entrance", "Front Exit", "Side Exit", "First Intermediate", "Second Intermediate"] ("Slit")
                    # "Set New Slit Positions"
                    n713 = call "JYSlits.vi"("JYMONOLib.IJYMonoReqd"=w1527, "Slit"=w1525, "error in (no error)"=w1526, "Slit Width"="Target\nFront Entrance") -> ("error out"=w1523:errorcluster)  [unwired: 1 in, 1 out]
                  }
                }
              }
            }
          }
        }
        n714 = local read "Close"() -> (w1465:bool)
      }
    }
  }
  n715 = flat-sequence {
    frame #0 {
      n716 = call <vilib>:"Create Report.vi"("window state (normal)"=T3."no change", "report type"=Report_Type."Excel", "template (empty)"=path "D:/desktop/train/TEST1/Save/2670中心波长.xlsx") -> ("report out"=w1534:refnum<class "NI_report.lvclass">, "error out"=w1533:errorcluster)  [unwired: 11 in]
      n717 = call-poly <vilib>:"Excel Get Data.vi"("report in"=w1534, "data type"=string[][] [], "error in (no error)"=w1533) -> ("report out"=w1529:refnum<class "NI_report.lvclass">, "data"=w1537:string[][], "error out"=w1528:errorcluster)  [unwired: 10 in]
      n718 = call-dynamic "Dispose Report.vi"("report in"=w1529, "error in (no error)"=w1528) -> ()  [unwired: 13 in, 1 out]
      n719 = Index Array(array=w1537, index (col)=0 ("禁用的索引 (列)")) -> (element=w1539:string[])  [unwired: 1 in]
      n720 = Fract/Exp String To Number(string=w1539) -> (number=→"波长范围":dbl[])  [unwired: 3 in, 1 out]
    }
  }
